vi "PTSAutoDaily.vi"() -> ()   [LabVIEW 2012]
uses:
  <vilib>/Utility/NIReport.llb/NI_report.lvclass
  <vilib>/addons/database/Connection.llb/DB Tools Open Connec (Path).vi
  <vilib>/addons/database/Connection.llb/Conn Execute.vi
  <vilib>/addons/database/Recordset.llb/Rec Fetch Recordset Data (R).vi
  <vilib>/addons/database/Recordset.llb/Rec Destroy - Connection.vi
  <vilib>/Utility/NIReport.llb/Append Text Table to Report (wrap).vi
  <vilib>/addons/database/_DB Variant To Data/Database Variant To Data.xnode
  <vilib>/addons/database/NI_Database_API.lvlib
  <vilib>/Utility/NIReport.llb/Excel/NI_Excel.lvclass
  <vilib>/addons/_office/NI_ReportGenerationToolkit.lvlib
panel:
  in  "Report Template":path=path "O:/Monitor/Report/PTSDailyReport.xls"
  in  "Table Control":string[][](table)
  in  "Table Control 2":string[][](table)
  in  "Table Control 3":string[][](table)
  in  "Table Control 4":string[][](table)
  out "error out 4":errorcluster
  out "error out 6":errorcluster
  out "appended array 5":string[](array[string])
  out "recordset data 5":variant[][](array[variant])
  out "error out 5":errorcluster
  out "appended array 4":string[](array[string])
  out "recordset data 4":variant[][](array[variant])
  out "error out 3":errorcluster
  out "appended array 3":string[](array[string])
  out "recordset data 3":variant[][](array[variant])
  out "error out":errorcluster
  out "appended array":string[](array[string])
  out "recordset data":variant[][](array[variant])
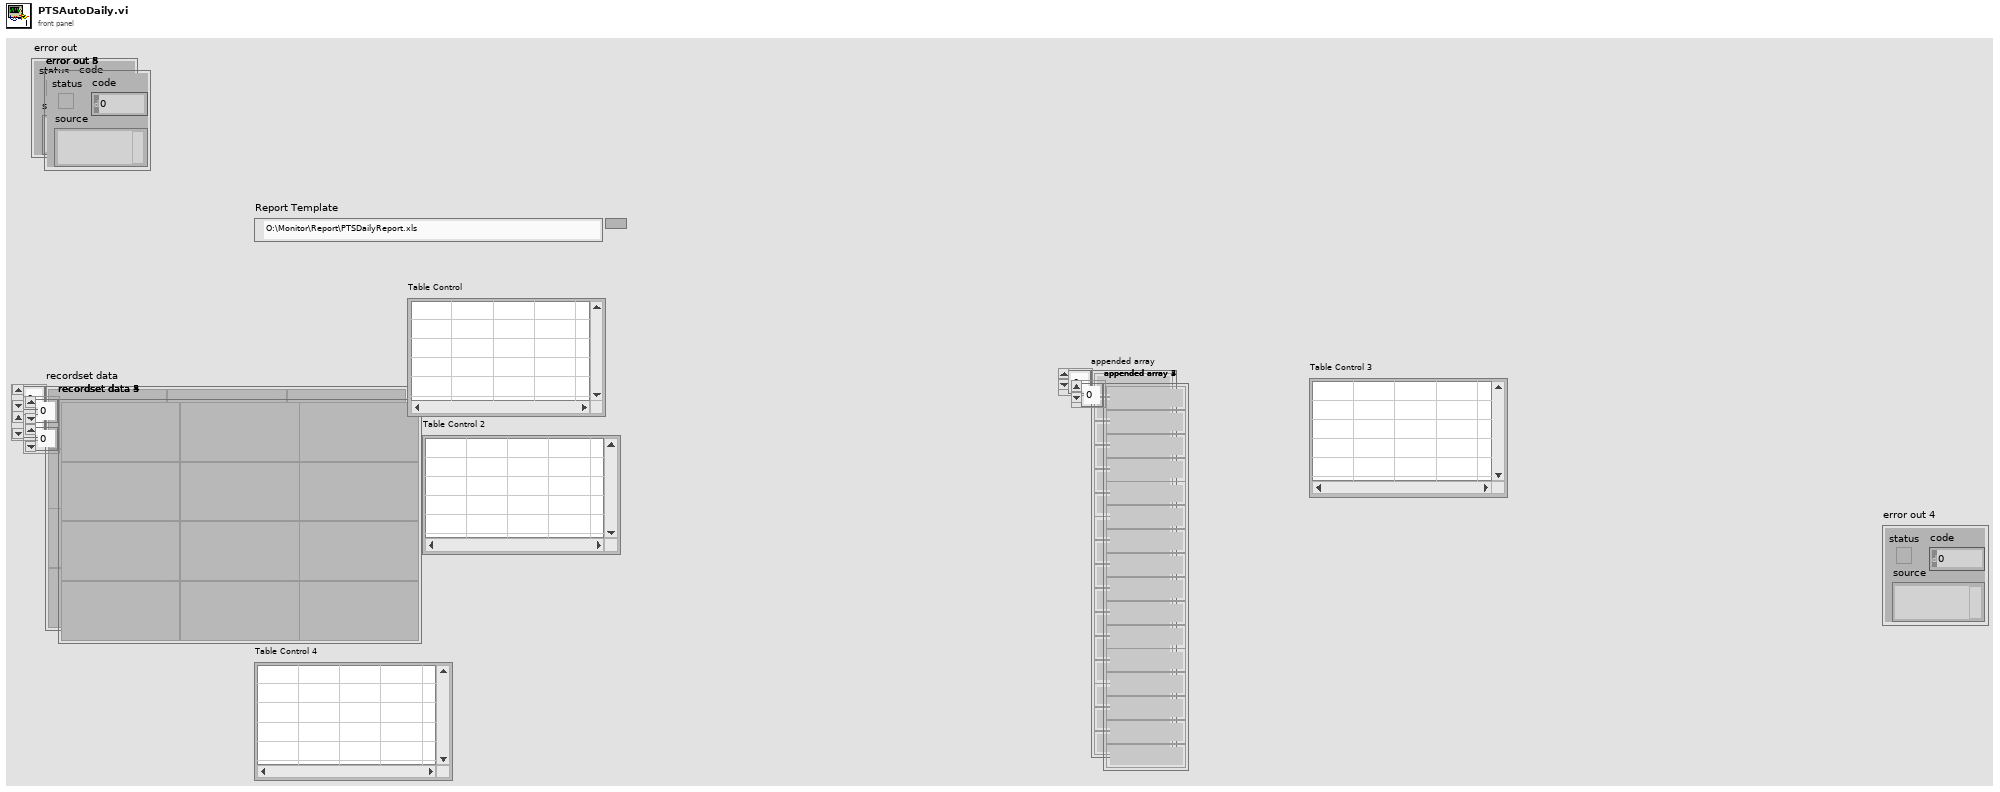
[diagram p1: front panel]
types:
  T1 = typedef "NI_Database_API.lvlib/Conn ObjectReference.ctl" = refnum<k1>
  T2 = typedef "NI_Database_API.lvlib/Rec ObjectReference.ctl" = refnum<k1>
  T3 = enum16{"Standard Report", "HTML", "Word", "Excel"}
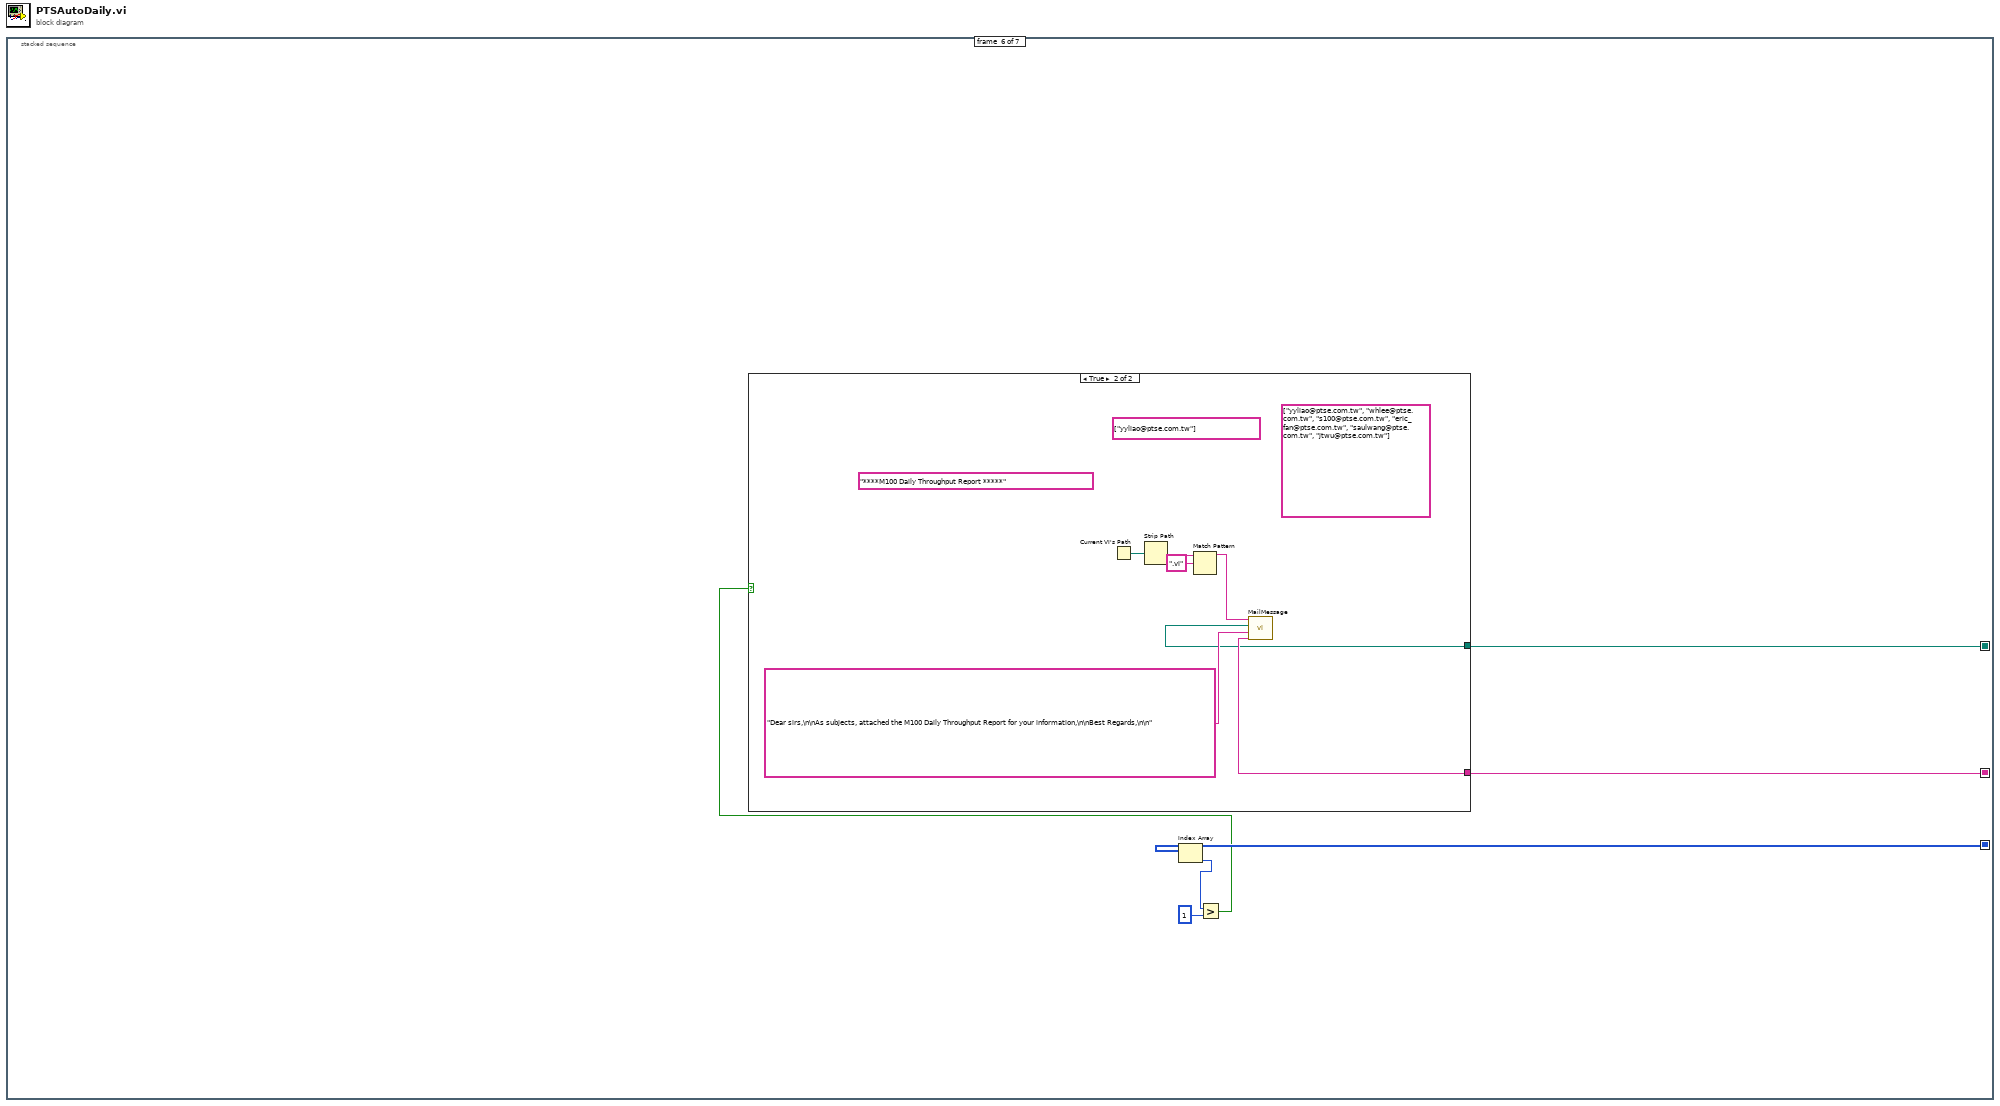
[diagram p0: block diagram]
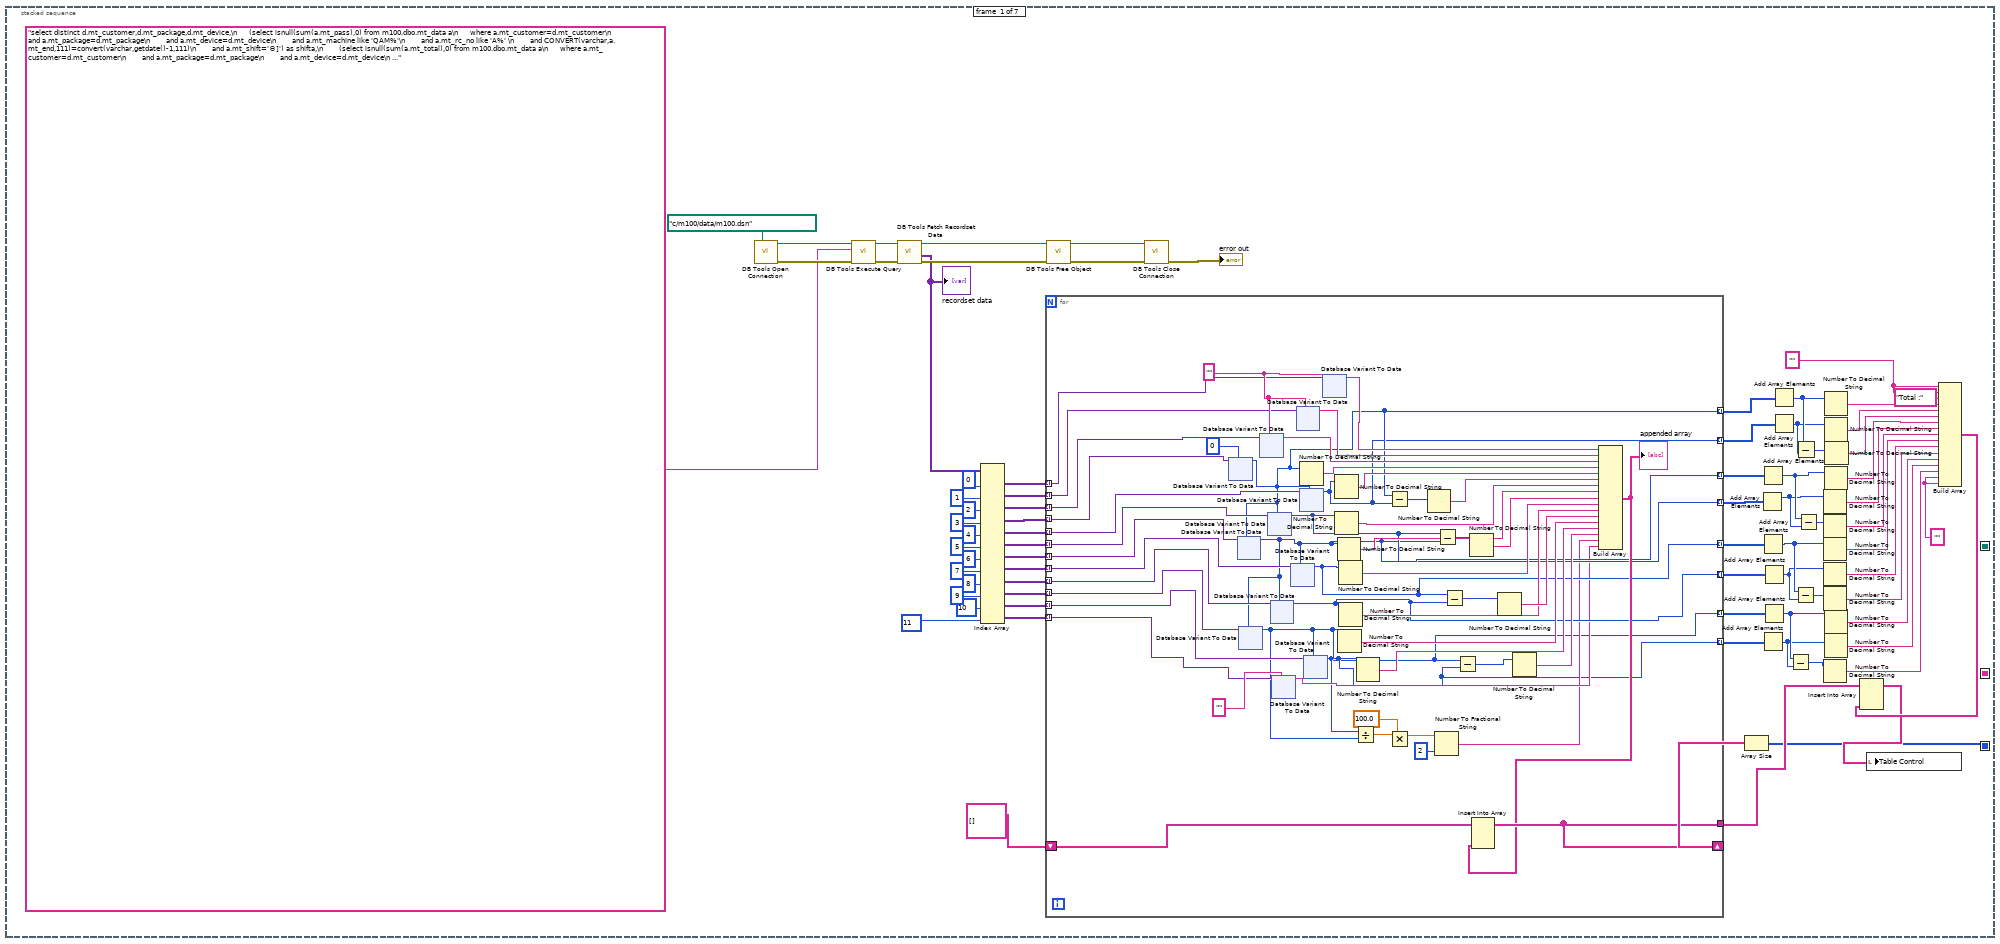
[diagram p2: hidden frame]
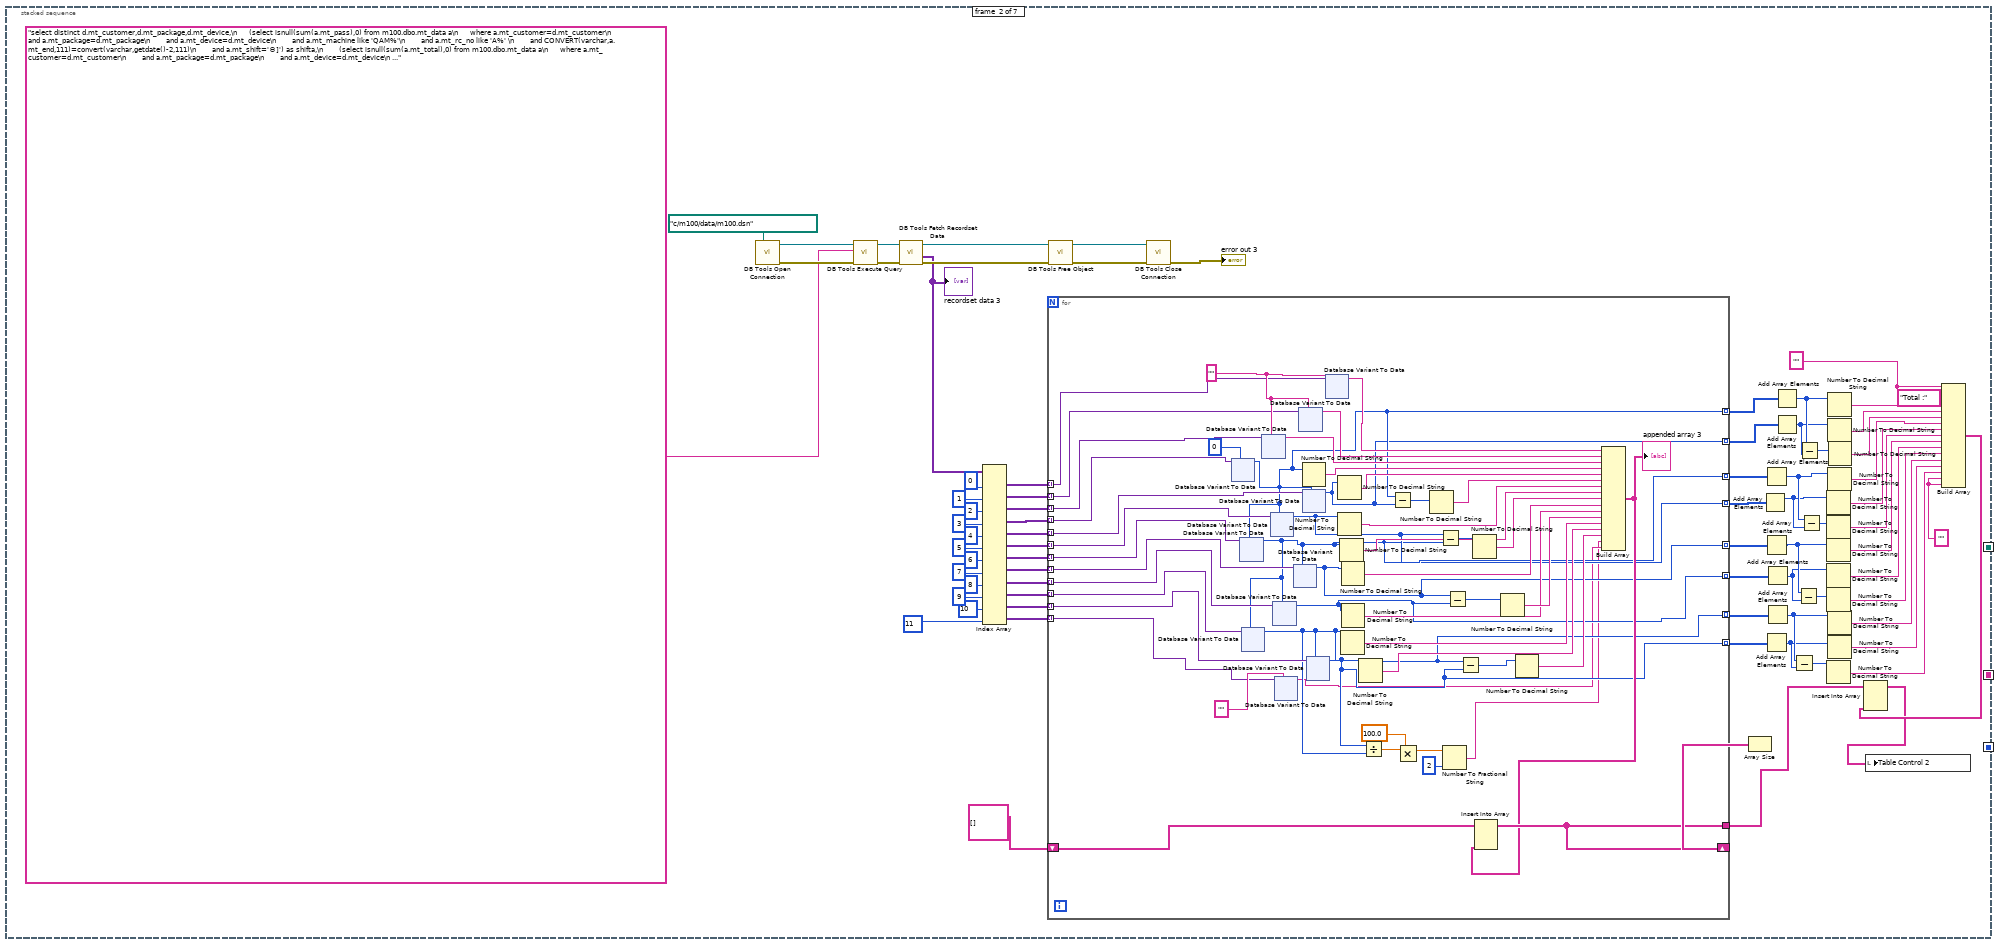
[diagram p3: hidden frame]
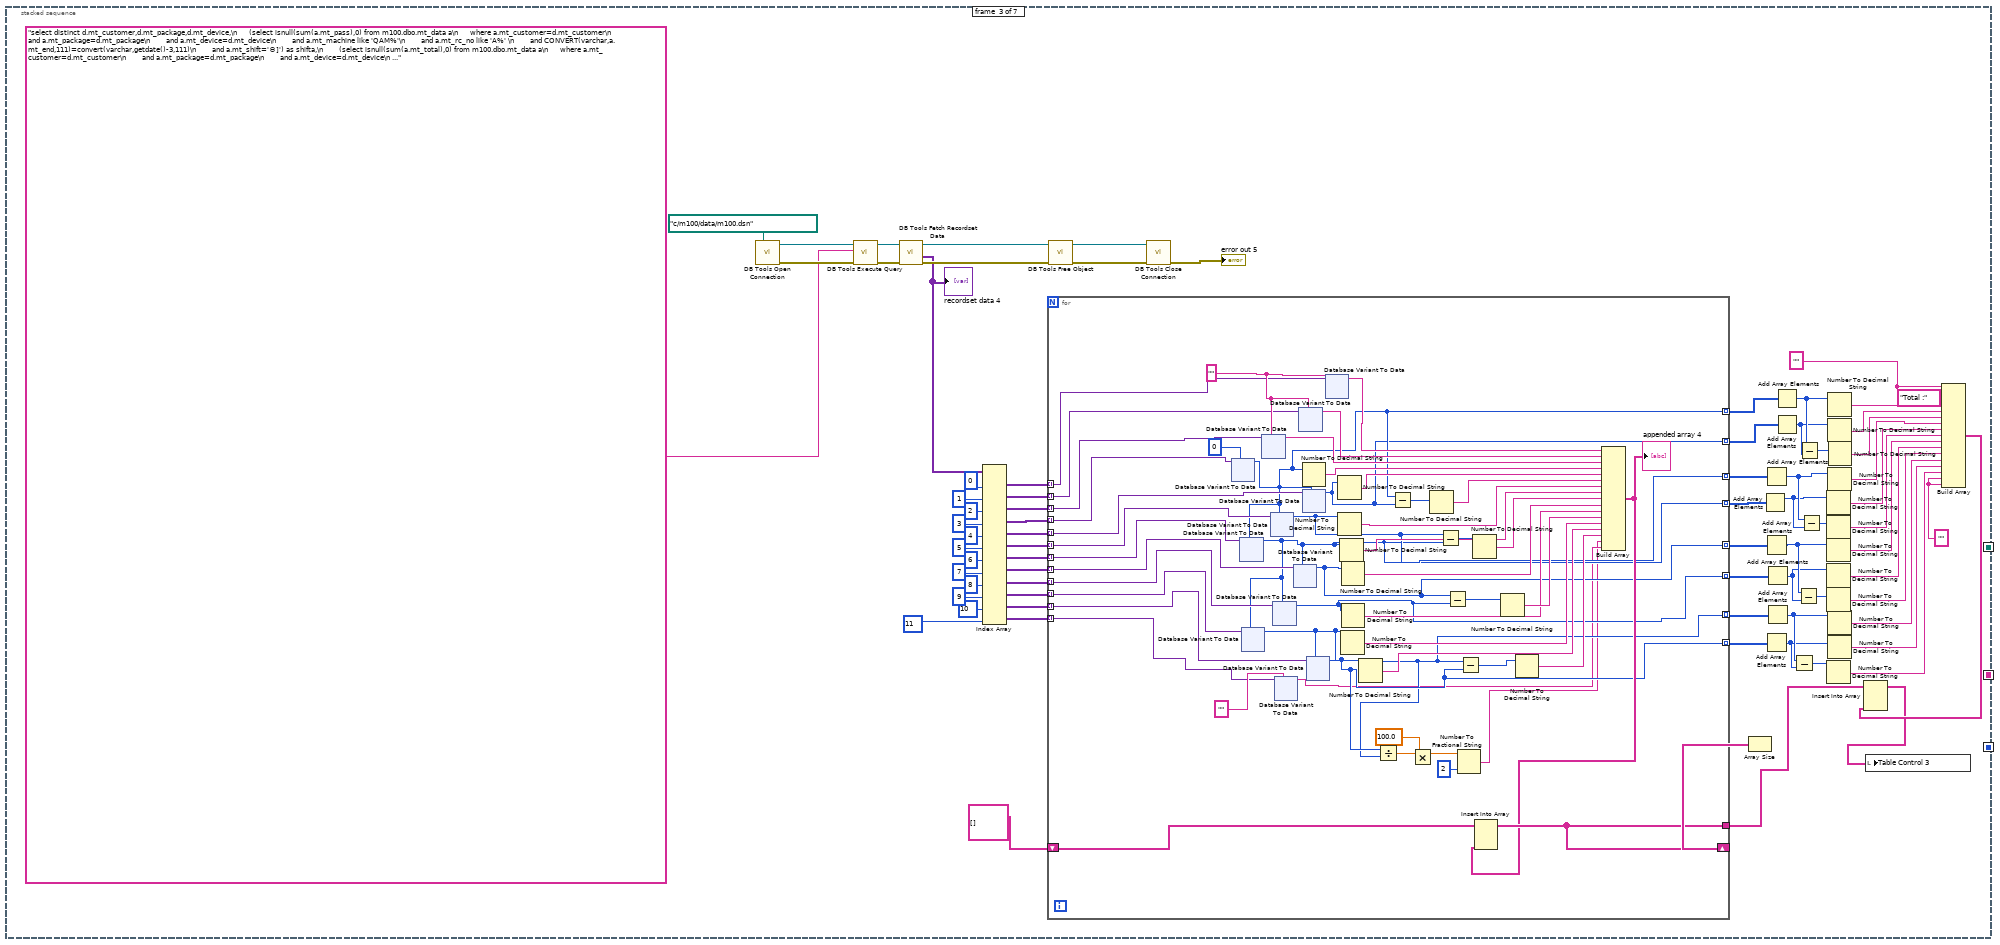
[diagram p4: hidden frame]
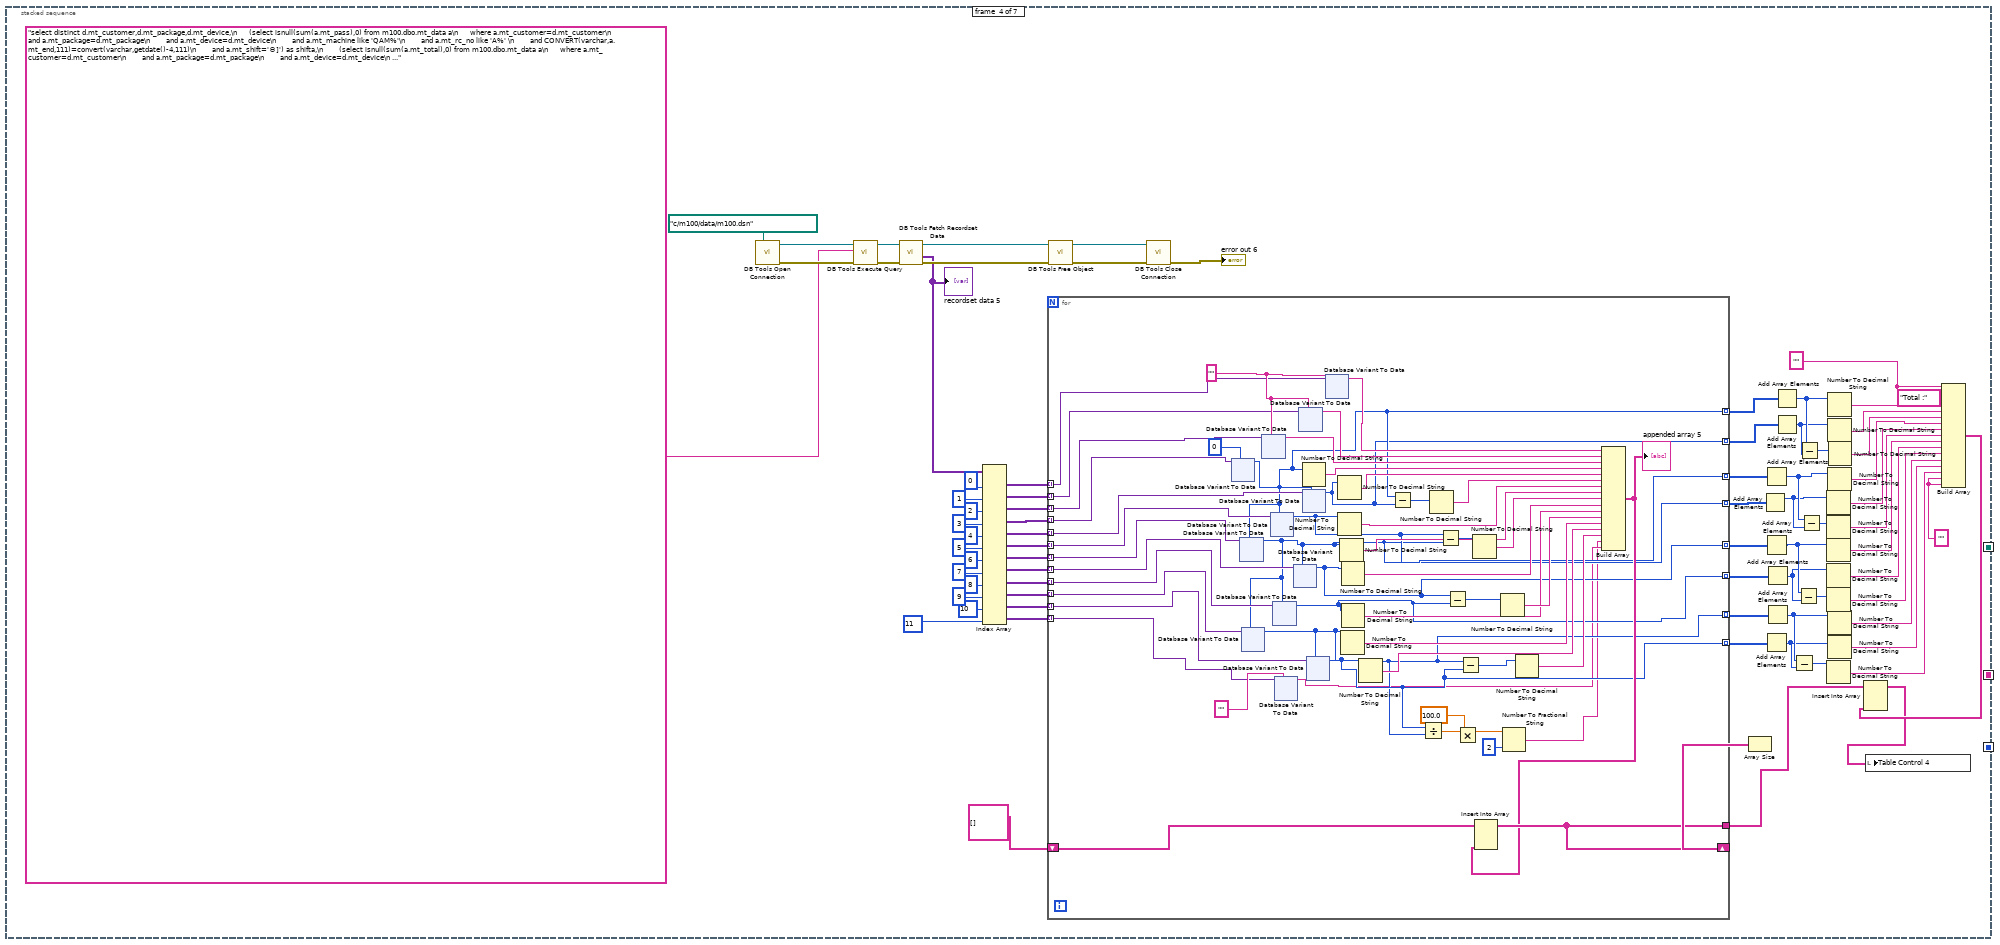
[diagram p5: hidden frame]
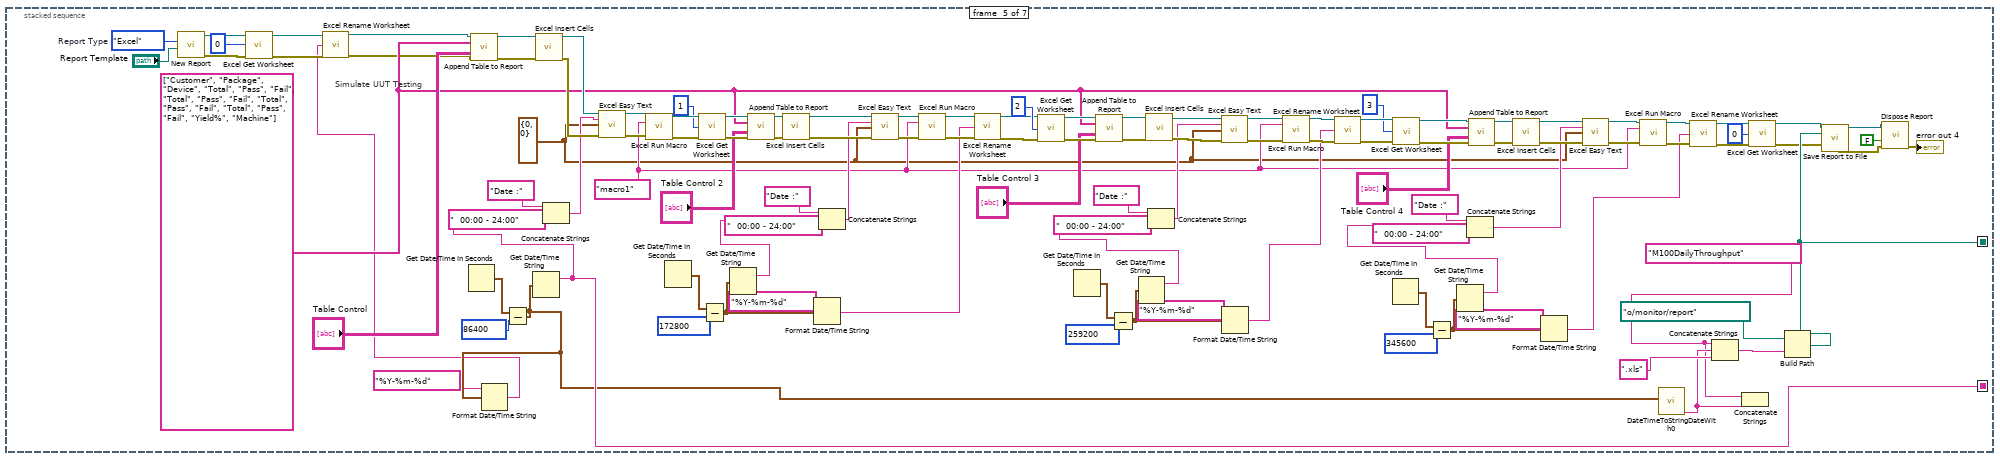
[diagram p6: hidden frame]
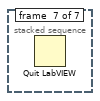
[diagram p8: hidden frame]
diagram:
  n1 = stacked-sequence {
    seq-local: [_ _ _ _ w2139 _ _] -> [_ _ _ _ _ w2163 _]
    seq-local: [_ _ _ _ w2138 _ _] -> [_ _ _ _ _ w2162 _]
    seq-local: [w2 _ _ _ _ _ _] -> [_ _ _ _ _ w2161 _]
    frame #0 {
      w1 = ""
      w37 = ""
      n2 = call-poly <vilib>:"DB Tools Open Connection.vi"("connection information"=path "c:/m100/data/m100.dsn") -> ("error out"=w72:errorcluster, "connection reference"=w76:T1)  [unwired: 7 in]
      n3 = call-poly <vilib>:"DB Tools Execute Query.vi"("error in (no error)"=w72, "SQL query"="select distinct d.mt_customer,d.mt_package,d.mt_device,\n      (select isnull(sum(a.mt_pass),0) from m100.dbo.mt_data a\n      where a.mt_customer=d.mt_customer\n        and a.mt_package=d.mt_package\n        and a.mt_device=d.mt_device\n        and a.mt_machine like 'QAM%'\n        and a.mt_rc_no like 'A%' \n        and CONVERT(varchar,a.mt_end,111)=convert(varchar,getdate()-1,111)\n        and a.mt_shift='©]') as shifta,\n        (select isnull(sum(a.mt_total),0) from m100.dbo.mt_data a\n      where a.mt_customer=d.mt_customer\n        and a.mt_package=d.mt_package\n        and a.mt_device=d.mt_device\n        and a.mt_machine like 'QAM%'\n        and a.mt_rc_no like 'A%' \n        and CONVERT(varchar,a.mt_end,111)=convert(varchar,getdate()-1,111)\n        and a.mt_shift='©]') as shifta1,\n        (select isnull(sum(b.mt_pass),0) from m100.dbo.mt_data b\n      where b.mt_customer=d.mt_customer\n        and b.mt_package=d.mt_package\n       and b.mt_device=d.mt_device\n        and b.mt_machine like 'QAM%'\n        and b.mt_rc_no like 'A%' \n        and CONVERT(varchar,b.mt_end,111)=convert(varchar,getdate()-1,111)\n        and b.mt_shift='¦­') as shiftb,\n        (select isnull(sum(b.mt_total),0) from m100.dbo.mt_data b\n      where b.mt_customer=d.mt_customer\n        and b.mt_package=d.mt_package\n        and b.mt_device=d.mt_device\n        and b.mt_machine like 'QAM%'\n        and b.mt_rc_no like 'A%' \n        and CONVERT(varchar,b.mt_end,111)=convert(varchar,getdate()-1,111)\n        and b.mt_shift='¦­') as shiftb1,\n        (select isnull(sum(c.mt_pass),0) from m100.dbo.mt_data c\n      where c.mt_customer=d.mt_customer\n        and c.mt_package=d.mt_package\n        and c.mt_device=d.mt_device\n        and c.mt_machine like 'QAM%'\n        and c.mt_rc_no like 'A%' \n        and CONVERT(varchar,c.mt_end,111)=convert(varchar,getdate()-1,111)\n        and c.mt_shift='¤¤') as shiftc,\n        (select isnull(sum(c.mt_total),0) from m100.dbo.mt_data c\n      where c.mt_customer=d.mt_customer\n        and c.mt_package=d.mt_package\n        and c.mt_device=d.mt_device\n        and c.mt_machine like 'QAM%'\n        and c.mt_rc_no like 'A%' \n        and CONVERT(varchar,c.mt_end,111)=convert(varchar,getdate()-1,111)\n        and c.mt_shift='¤¤') as shiftc1,\n        SUM(mt_pass),SUM(mt_total),master.dbo.GetEntityNameFromDateToDate(d.mt_customer,d.mt_package,d.mt_device,CONVERT(varchar,GETDATE()-1,111),CONVERT(varchar,GETDATE()-1,111))\n  FROM [m100].[dbo].[mt_data] d\n  WHERE d.mt_machine like 'QAM%'\n    AND CONVERT(varchar,d.mt_end,111)=convert(varchar,getdate()-1,111)\n    and d.mt_pass > 0 and d.mt_rc_no like 'A%'\n      group by d.mt_customer,d.mt_package,d.mt_device", "connection reference"=w76) -> ("error out"=w71:errorcluster, "recordset reference"=w75:T2)  [unwired: 5 in]
      n4 = call-poly <vilib>:"DB Tools Fetch Recordset Data.vi"("error in (no error)"=w71, "recordset reference"=w75) -> ("error out"=w70:errorcluster, "recordset data"=w40:variant[][], "recordset reference out"=w74:T2)  [unwired: 3 in]
      "recordset data" <- w40
      n5 = Index Array(array=w40, index (col) #1=0 ("index (row)"), index (col) #2=1 ("index (col)"), index (col) #3=2 ("disabled index (col)"), index (col) #4=3 ("index (col)"), index (col) #5=4 ("index (col)"), index (col) #6=5 ("index (col)"), index (col) #7=6 ("index (col)"), index (col) #8=7 ("index (col)"), index (col) #9=8 ("index (col)"), index (col) #10=9 ("index (col)"), index (col) #11=10 ("index (col)"), index (col) #12=11 ("index (col)")) -> (element #1=w44:variant[], element #2=w43:variant[], element #3=w57:variant[], element #4=w56:variant[], element #5=w55:variant[], element #6=w54:variant[], element #7=w53:variant[], element #8=w52:variant[], element #9=w51:variant[], element #10=w50:variant[], element #11=w49:variant[], element #12=w48:variant[])  [unwired: 12 in]
      n6 = for {
        tunnel: w57 -> [w102] mode=indexing
        tunnel: w56 -> [w101] mode=indexing
        tunnel: w55 -> [w100] mode=indexing
        tunnel: w54 -> [w99] mode=indexing
        tunnel: w53 -> [w98] mode=indexing
        tunnel: w52 -> [w97] mode=indexing
        tunnel: w51 -> [w96] mode=indexing
        tunnel: w50 -> [w95] mode=indexing
        tunnel: w49 -> [w94] mode=indexing
        tunnel: w48 -> [w93] mode=indexing
        tunnel: [w128] -> w30
        shift-right: [w128] -> w46
        shift-left: string[][] [] ("array") -> [w127]
        tunnel: w44 -> [w104] mode=indexing
        tunnel: w43 -> [w103] mode=indexing
        tunnel: [w91] -> w39 mode=indexing
        tunnel: [w90] -> w38 mode=indexing
        tunnel: [w89] -> w28 mode=indexing
        tunnel: [w88] -> w27 mode=indexing
        tunnel: [w87] -> w19 mode=indexing
        tunnel: [w86] -> w18 mode=indexing
        tunnel: [w78] -> w11 mode=indexing
        tunnel: [w79] -> w10 mode=indexing
        w126 = ""
        n7 = xnode "Database Variant To Data"("database variant"=w101, "type"=0) -> ("data"=w91:i32)  [unwired: 1 in, 1 out]
        n8 = xnode "Database Variant To Data"("database variant"=w98, "type"=w91) -> ("data"=w88:i32)  [unwired: 1 in, 1 out]
        n9 = xnode "Database Variant To Data"("database variant"=w95, "type"=w88) -> ("data"=w78:i32)  [unwired: 1 in, 1 out]
        n10 = xnode "Database Variant To Data"("database variant"=w102, "type"=w126) -> ("data"=w110:string)  [unwired: 1 in, 1 out]
        n11 = xnode "Database Variant To Data"("database variant"=w99, "type"=w91) -> ("data"=w89:i32)  [unwired: 1 in, 1 out]
        n12 = xnode "Database Variant To Data"("database variant"=w96, "type"=w88) -> ("data"=w86:i32)  [unwired: 1 in, 1 out]
        n13 = xnode "Database Variant To Data"("database variant"=w93, "type"="") -> ("data"=w81:string)  [unwired: 1 in, 1 out]
        n14 = xnode "Database Variant To Data"("database variant"=w97, "type"=w88) -> ("data"=w87:i32)  [unwired: 1 in, 1 out]
        n15 = xnode "Database Variant To Data"("database variant"=w103, "type"=w126) -> ("data"=w107:string)  [unwired: 1 in, 1 out]
        n16 = Number To Decimal String(number=w91) -> (decimal integer string=w109:string)  [unwired: 1 in]
        n17 = xnode "Database Variant To Data"("database variant"=w100, "type"=w91) -> ("data"=w90:i32)  [unwired: 1 in, 1 out]
        n18 = xnode "Database Variant To Data"("database variant"=w94, "type"=w78) -> ("data"=w79:i32)  [unwired: 1 in, 1 out]
        n19 = xnode "Database Variant To Data"("database variant"=w104, "type"=w126) -> ("data"=w111:string)  [unwired: 1 in, 1 out]
        n20 = Number To Decimal String(number=w90) -> (decimal integer string=w108:string)  [unwired: 1 in]
        n21 = Number To Decimal String(number=w89) -> (decimal integer string=w124:string)  [unwired: 1 in]
        n22 = Number To Decimal String(number=w88) -> (decimal integer string=w123:string)  [unwired: 1 in]
        n23 = Number To Decimal String(number=w78) -> (decimal integer string=w118:string)  [unwired: 1 in]
        n24 = Number To Decimal String(number=w87) -> (decimal integer string=w114:string)  [unwired: 1 in]
        n25 = Number To Decimal String(number=w86) -> (decimal integer string=w115:string)  [unwired: 1 in]
        n26 = Divide(x=w79, y=w78) -> (x/y=w85:dbl)
        n27 = Number To Decimal String(number=w79) -> (decimal integer string=w119:string)  [unwired: 1 in]
        n28 = Subtract(x=w91, y=w90) -> (x-y=w106:i32)
        n29 = Multiply(x=w85, y=100.0) -> (x*y=w83:dbl)
        n30 = Number To Decimal String(number=w106) -> (decimal integer string=w105:string)  [unwired: 1 in]
        n31 = Number To Fractional String(number=w83, precision (6)=i16 2) -> (F-format string=w80:string)  [unwired: 2 in]
        n32 = Subtract(x=w89, y=w88) -> (x-y=w113:i32)
        n33 = Subtract(x=w87, y=w86) -> (x-y=w117:i32)
        n34 = Subtract(x=w78, y=w79) -> (x-y=w121:i32)
        n35 = Number To Decimal String(number=w113) -> (decimal integer string=w112:string)  [unwired: 1 in]
        n36 = Number To Decimal String(number=w117) -> (decimal integer string=w116:string)  [unwired: 1 in]
        n37 = Number To Decimal String(number=w121) -> (decimal integer string=w120:string)  [unwired: 1 in]
        n38 = Build Array(w111, w107, w110, w109, w108, w105, w124, w123, w112, w114, w115, w116, w118, w119, w120, w80, w81) -> (w92:string[])
        "appended array" <- w92
        n39 = Insert Into Array(array=w127, new element=w92) -> (w128:string[][])  [unwired: 2 in]
      }
      n40 = call-poly <vilib>:"DB Tools Free Object.vi"("error in (no error)"=w70, "recordset reference"=w74) -> ("error out"=w69:errorcluster, "connection reference"=w73:T1)  [unwired: 8 in]
      n41 = call <vilib>:"DB Tools Close Connection.vi"("error in (no error)"=w69, "connection reference"=w73) -> ("error out"=→"error out":errorcluster)  [unwired: 5 in]
      n42 = Array Size(array=w46) -> (size(s)=w2:i32[])
      n43 = Add Array Elements(numeric array=w27) -> (sum=w22:i32)
      n44 = Add Array Elements(numeric array=w28) -> (sum=w23:i32)
      n45 = Add Array Elements(numeric array=w19) -> (sum=w15:i32)
      n46 = Add Array Elements(numeric array=w10) -> (sum=w8:i32)
      n47 = Add Array Elements(numeric array=w18) -> (sum=w14:i32)
      n48 = Add Array Elements(numeric array=w11) -> (sum=w9:i32)
      n49 = Add Array Elements(numeric array=w39) -> (sum=w34:i32)
      n50 = Add Array Elements(numeric array=w38) -> (sum=w33:i32)
      n51 = Subtract(x=w9, y=w8) -> (x-y=w7:i32)
      n52 = Subtract(x=w15, y=w14) -> (x-y=w12:i32)
      n53 = Subtract(x=w34, y=w33) -> (x-y=w26:i32)
      n54 = Subtract(x=w23, y=w22) -> (x-y=w20:i32)
      n55 = Number To Decimal String(number=w22) -> (decimal integer string=w24:string)  [unwired: 1 in]
      n56 = Number To Decimal String(number=w20) -> (decimal integer string=w21:string)  [unwired: 1 in]
      n57 = Number To Decimal String(number=w15) -> (decimal integer string=w17:string)  [unwired: 1 in]
      n58 = Number To Decimal String(number=w14) -> (decimal integer string=w16:string)  [unwired: 1 in]
      n59 = Number To Decimal String(number=w12) -> (decimal integer string=w13:string)  [unwired: 1 in]
      n60 = Number To Decimal String(number=w7) -> (decimal integer string=w4:string)  [unwired: 1 in]
      n61 = Number To Decimal String(number=w34) -> (decimal integer string=w36:string)  [unwired: 1 in]
      n62 = Number To Decimal String(number=w33) -> (decimal integer string=w35:string)  [unwired: 1 in]
      n63 = Number To Decimal String(number=w23) -> (decimal integer string=w25:string)  [unwired: 1 in]
      n64 = Number To Decimal String(number=w9) -> (decimal integer string=w6:string)  [unwired: 1 in]
      n65 = Number To Decimal String(number=w8) -> (decimal integer string=w5:string)  [unwired: 1 in]
      n66 = Number To Decimal String(number=w26) -> (decimal integer string=w32:string)  [unwired: 1 in]
      n67 = Build Array(w37, w37, "Total :" ("element"), w36, w35, w32, w25, w24, w21, w17, w16, w13, w6, w5, w4, w1, w1) -> (w31:string[])
      n68 = Insert Into Array(array=w30, new element=w31) -> (w29:string[][])  [unwired: 2 in]
      n69 = local write "Table Control"(w29) -> ()
    }
    frame #1 {
      w513 = ""
      w548 = ""
      n70 = call-poly <vilib>:"DB Tools Open Connection.vi"("connection information"=path "c:/m100/data/m100.dsn") -> ("error out"=w583:errorcluster, "connection reference"=w587:T1)  [unwired: 7 in]
      n71 = call-poly <vilib>:"DB Tools Execute Query.vi"("error in (no error)"=w583, "SQL query"="select distinct d.mt_customer,d.mt_package,d.mt_device,\n      (select isnull(sum(a.mt_pass),0) from m100.dbo.mt_data a\n      where a.mt_customer=d.mt_customer\n        and a.mt_package=d.mt_package\n        and a.mt_device=d.mt_device\n        and a.mt_machine like 'QAM%'\n        and a.mt_rc_no like 'A%' \n        and CONVERT(varchar,a.mt_end,111)=convert(varchar,getdate()-2,111)\n        and a.mt_shift='©]') as shifta,\n        (select isnull(sum(a.mt_total),0) from m100.dbo.mt_data a\n      where a.mt_customer=d.mt_customer\n        and a.mt_package=d.mt_package\n        and a.mt_device=d.mt_device\n        and a.mt_machine like 'QAM%'\n        and a.mt_rc_no like 'A%' \n        and CONVERT(varchar,a.mt_end,111)=convert(varchar,getdate()-2,111)\n        and a.mt_shift='©]') as shifta1,\n        (select isnull(sum(b.mt_pass),0) from m100.dbo.mt_data b\n      where b.mt_customer=d.mt_customer\n        and b.mt_package=d.mt_package\n       and b.mt_device=d.mt_device\n        and b.mt_machine like 'QAM%'\n        and b.mt_rc_no like 'A%' \n        and CONVERT(varchar,b.mt_end,111)=convert(varchar,getdate()-2,111)\n        and b.mt_shift='¦­') as shiftb,\n        (select isnull(sum(b.mt_total),0) from m100.dbo.mt_data b\n      where b.mt_customer=d.mt_customer\n        and b.mt_package=d.mt_package\n        and b.mt_device=d.mt_device\n        and b.mt_machine like 'QAM%'\n        and b.mt_rc_no like 'A%' \n        and CONVERT(varchar,b.mt_end,111)=convert(varchar,getdate()-2,111)\n        and b.mt_shift='¦­') as shiftb1,\n        (select isnull(sum(c.mt_pass),0) from m100.dbo.mt_data c\n      where c.mt_customer=d.mt_customer\n        and c.mt_package=d.mt_package\n        and c.mt_device=d.mt_device\n        and c.mt_machine like 'QAM%'\n        and c.mt_rc_no like 'A%' \n        and CONVERT(varchar,c.mt_end,111)=convert(varchar,getdate()-2,111)\n        and c.mt_shift='¤¤') as shiftc,\n        (select isnull(sum(c.mt_total),0) from m100.dbo.mt_data c\n      where c.mt_customer=d.mt_customer\n        and c.mt_package=d.mt_package\n        and c.mt_device=d.mt_device\n        and c.mt_machine like 'QAM%'\n        and c.mt_rc_no like 'A%' \n        and CONVERT(varchar,c.mt_end,111)=convert(varchar,getdate()-2,111)\n        and c.mt_shift='¤¤') as shiftc1,\n        SUM(mt_pass),SUM(mt_total),master.dbo.GetEntityNameFromDateToDate(d.mt_customer,d.mt_package,d.mt_device,CONVERT(varchar,GETDATE()-2,111),CONVERT(varchar,GETDATE()-2,111))\n  FROM [m100].[dbo].[mt_data] d\n  WHERE  d.mt_machine like 'QAM%'\n    AND CONVERT(varchar,d.mt_end,111)=convert(varchar,getdate()-2,111)\n    and d.mt_pass > 0 and d.mt_rc_no like 'A%'\n      group by d.mt_customer,d.mt_package,d.mt_device", "connection reference"=w587) -> ("error out"=w582:errorcluster, "recordset reference"=w586:T2)  [unwired: 5 in]
      n72 = call-poly <vilib>:"DB Tools Fetch Recordset Data.vi"("error in (no error)"=w582, "recordset reference"=w586) -> ("error out"=w581:errorcluster, "recordset data"=w551:variant[][], "recordset reference out"=w585:T2)  [unwired: 3 in]
      "recordset data 3" <- w551
      n73 = Index Array(array=w551, index (col) #1=0 ("index (row)"), index (col) #2=1 ("index (col)"), index (col) #3=2 ("disabled index (col)"), index (col) #4=3 ("index (col)"), index (col) #5=4 ("index (col)"), index (col) #6=5 ("index (col)"), index (col) #7=6 ("index (col)"), index (col) #8=7 ("index (col)"), index (col) #9=8 ("index (col)"), index (col) #10=9 ("index (col)"), index (col) #11=10 ("index (col)"), index (col) #12=11 ("index (col)")) -> (element #1=w555:variant[], element #2=w554:variant[], element #3=w568:variant[], element #4=w567:variant[], element #5=w566:variant[], element #6=w565:variant[], element #7=w564:variant[], element #8=w563:variant[], element #9=w562:variant[], element #10=w561:variant[], element #11=w560:variant[], element #12=w559:variant[])  [unwired: 12 in]
      n74 = for {
        tunnel: w568 -> [w613] mode=indexing
        tunnel: w567 -> [w612] mode=indexing
        tunnel: w566 -> [w611] mode=indexing
        tunnel: w565 -> [w610] mode=indexing
        tunnel: w564 -> [w609] mode=indexing
        tunnel: w563 -> [w608] mode=indexing
        tunnel: w562 -> [w607] mode=indexing
        tunnel: w561 -> [w606] mode=indexing
        tunnel: w560 -> [w605] mode=indexing
        tunnel: w559 -> [w604] mode=indexing
        tunnel: [w639] -> w541
        shift-right: [w639] -> w557
        shift-left: string[][] [] ("array") -> [w638]
        tunnel: w555 -> [w615] mode=indexing
        tunnel: w554 -> [w614] mode=indexing
        tunnel: [w602] -> w550 mode=indexing
        tunnel: [w601] -> w549 mode=indexing
        tunnel: [w600] -> w539 mode=indexing
        tunnel: [w599] -> w538 mode=indexing
        tunnel: [w598] -> w530 mode=indexing
        tunnel: [w597] -> w529 mode=indexing
        tunnel: [w591] -> w522 mode=indexing
        tunnel: [w592] -> w521 mode=indexing
        w637 = ""
        n75 = xnode "Database Variant To Data"("database variant"=w612, "type"=0) -> ("data"=w602:i32)  [unwired: 1 in, 1 out]
        n76 = xnode "Database Variant To Data"("database variant"=w609, "type"=w602) -> ("data"=w599:i32)  [unwired: 1 in, 1 out]
        n77 = xnode "Database Variant To Data"("database variant"=w606, "type"=w599) -> ("data"=w591:i32)  [unwired: 1 in, 1 out]
        n78 = xnode "Database Variant To Data"("database variant"=w613, "type"=w637) -> ("data"=w621:string)  [unwired: 1 in, 1 out]
        n79 = xnode "Database Variant To Data"("database variant"=w610, "type"=w602) -> ("data"=w600:i32)  [unwired: 1 in, 1 out]
        n80 = xnode "Database Variant To Data"("database variant"=w607, "type"=w599) -> ("data"=w597:i32)  [unwired: 1 in, 1 out]
        n81 = xnode "Database Variant To Data"("database variant"=w604, "type"="") -> ("data"=w590:string)  [unwired: 1 in, 1 out]
        n82 = xnode "Database Variant To Data"("database variant"=w608, "type"=w599) -> ("data"=w598:i32)  [unwired: 1 in, 1 out]
        n83 = xnode "Database Variant To Data"("database variant"=w614, "type"=w637) -> ("data"=w618:string)  [unwired: 1 in, 1 out]
        n84 = Number To Decimal String(number=w602) -> (decimal integer string=w620:string)  [unwired: 1 in]
        n85 = xnode "Database Variant To Data"("database variant"=w611, "type"=w602) -> ("data"=w601:i32)  [unwired: 1 in, 1 out]
        n86 = xnode "Database Variant To Data"("database variant"=w605, "type"=w591) -> ("data"=w592:i32)  [unwired: 1 in, 1 out]
        n87 = xnode "Database Variant To Data"("database variant"=w615, "type"=w637) -> ("data"=w622:string)  [unwired: 1 in, 1 out]
        n88 = Number To Decimal String(number=w601) -> (decimal integer string=w619:string)  [unwired: 1 in]
        n89 = Number To Decimal String(number=w600) -> (decimal integer string=w635:string)  [unwired: 1 in]
        n90 = Number To Decimal String(number=w599) -> (decimal integer string=w634:string)  [unwired: 1 in]
        n91 = Number To Decimal String(number=w591) -> (decimal integer string=w629:string)  [unwired: 1 in]
        n92 = Number To Decimal String(number=w598) -> (decimal integer string=w625:string)  [unwired: 1 in]
        n93 = Number To Decimal String(number=w597) -> (decimal integer string=w626:string)  [unwired: 1 in]
        n94 = Number To Decimal String(number=w592) -> (decimal integer string=w630:string)  [unwired: 1 in]
        n95 = Divide(x=w592, y=w591) -> (x/y=w596:dbl)
        n96 = Subtract(x=w602, y=w601) -> (x-y=w617:i32)
        n97 = Multiply(x=w596, y=100.0) -> (x*y=w594:dbl)
        n98 = Number To Decimal String(number=w617) -> (decimal integer string=w616:string)  [unwired: 1 in]
        n99 = Subtract(x=w600, y=w599) -> (x-y=w624:i32)
        n100 = Number To Fractional String(number=w594, precision (6)=i16 2) -> (F-format string=w589:string)  [unwired: 2 in]
        n101 = Subtract(x=w598, y=w597) -> (x-y=w628:i32)
        n102 = Subtract(x=w591, y=w592) -> (x-y=w632:i32)
        n103 = Number To Decimal String(number=w624) -> (decimal integer string=w623:string)  [unwired: 1 in]
        n104 = Number To Decimal String(number=w628) -> (decimal integer string=w627:string)  [unwired: 1 in]
        n105 = Number To Decimal String(number=w632) -> (decimal integer string=w631:string)  [unwired: 1 in]
        n106 = Build Array(w622, w618, w621, w620, w619, w616, w635, w634, w623, w625, w626, w627, w629, w630, w631, w589, w590) -> (w603:string[])
        "appended array 3" <- w603
        n107 = Insert Into Array(array=w638, new element=w603) -> (w639:string[][])  [unwired: 2 in]
      }
      n108 = call-poly <vilib>:"DB Tools Free Object.vi"("error in (no error)"=w581, "recordset reference"=w585) -> ("error out"=w580:errorcluster, "connection reference"=w584:T1)  [unwired: 8 in]
      n109 = call <vilib>:"DB Tools Close Connection.vi"("error in (no error)"=w580, "connection reference"=w584) -> ("error out"=→"error out 3":errorcluster)  [unwired: 5 in]
      n110 = Array Size(array=w557) -> ()  [unwired: 1 out]
      n111 = Add Array Elements(numeric array=w538) -> (sum=w533:i32)
      n112 = Add Array Elements(numeric array=w539) -> (sum=w534:i32)
      n113 = Add Array Elements(numeric array=w530) -> (sum=w526:i32)
      n114 = Add Array Elements(numeric array=w521) -> (sum=w519:i32)
      n115 = Add Array Elements(numeric array=w529) -> (sum=w525:i32)
      n116 = Add Array Elements(numeric array=w522) -> (sum=w520:i32)
      n117 = Add Array Elements(numeric array=w550) -> (sum=w545:i32)
      n118 = Add Array Elements(numeric array=w549) -> (sum=w544:i32)
      n119 = Subtract(x=w520, y=w519) -> (x-y=w518:i32)
      n120 = Subtract(x=w526, y=w525) -> (x-y=w523:i32)
      n121 = Subtract(x=w545, y=w544) -> (x-y=w537:i32)
      n122 = Subtract(x=w534, y=w533) -> (x-y=w531:i32)
      n123 = Number To Decimal String(number=w533) -> (decimal integer string=w535:string)  [unwired: 1 in]
      n124 = Number To Decimal String(number=w531) -> (decimal integer string=w532:string)  [unwired: 1 in]
      n125 = Number To Decimal String(number=w526) -> (decimal integer string=w528:string)  [unwired: 1 in]
      n126 = Number To Decimal String(number=w525) -> (decimal integer string=w527:string)  [unwired: 1 in]
      n127 = Number To Decimal String(number=w523) -> (decimal integer string=w524:string)  [unwired: 1 in]
      n128 = Number To Decimal String(number=w518) -> (decimal integer string=w515:string)  [unwired: 1 in]
      n129 = Number To Decimal String(number=w545) -> (decimal integer string=w547:string)  [unwired: 1 in]
      n130 = Number To Decimal String(number=w544) -> (decimal integer string=w546:string)  [unwired: 1 in]
      n131 = Number To Decimal String(number=w534) -> (decimal integer string=w536:string)  [unwired: 1 in]
      n132 = Number To Decimal String(number=w520) -> (decimal integer string=w517:string)  [unwired: 1 in]
      n133 = Number To Decimal String(number=w519) -> (decimal integer string=w516:string)  [unwired: 1 in]
      n134 = Number To Decimal String(number=w537) -> (decimal integer string=w543:string)  [unwired: 1 in]
      n135 = Build Array(w548, w548, "Total :" ("element"), w547, w546, w543, w536, w535, w532, w528, w527, w524, w517, w516, w515, w513, w513) -> (w542:string[])
      n136 = Insert Into Array(array=w541, new element=w542) -> (w540:string[][])  [unwired: 2 in]
      n137 = local write "Table Control 2"(w540) -> ()
    }
    frame #2 {
      w1024 = ""
      w1059 = ""
      n138 = call-poly <vilib>:"DB Tools Open Connection.vi"("connection information"=path "c:/m100/data/m100.dsn") -> ("error out"=w1094:errorcluster, "connection reference"=w1098:T1)  [unwired: 7 in]
      n139 = call-poly <vilib>:"DB Tools Execute Query.vi"("error in (no error)"=w1094, "SQL query"="select distinct d.mt_customer,d.mt_package,d.mt_device,\n      (select isnull(sum(a.mt_pass),0) from m100.dbo.mt_data a\n      where a.mt_customer=d.mt_customer\n        and a.mt_package=d.mt_package\n        and a.mt_device=d.mt_device\n        and a.mt_machine like 'QAM%'\n        and a.mt_rc_no like 'A%' \n        and CONVERT(varchar,a.mt_end,111)=convert(varchar,getdate()-3,111)\n        and a.mt_shift='©]') as shifta,\n        (select isnull(sum(a.mt_total),0) from m100.dbo.mt_data a\n      where a.mt_customer=d.mt_customer\n        and a.mt_package=d.mt_package\n        and a.mt_device=d.mt_device\n        and a.mt_machine like 'QAM%'\n        and a.mt_rc_no like 'A%' \n        and CONVERT(varchar,a.mt_end,111)=convert(varchar,getdate()-3,111)\n        and a.mt_shift='©]') as shifta1,\n        (select isnull(sum(b.mt_pass),0) from m100.dbo.mt_data b\n      where b.mt_customer=d.mt_customer\n        and b.mt_package=d.mt_package\n       and b.mt_device=d.mt_device\n        and b.mt_machine like 'QAM%'\n        and b.mt_rc_no like 'A%' \n        and CONVERT(varchar,b.mt_end,111)=convert(varchar,getdate()-3,111)\n        and b.mt_shift='¦­') as shiftb,\n        (select isnull(sum(b.mt_total),0) from m100.dbo.mt_data b\n      where b.mt_customer=d.mt_customer\n        and b.mt_package=d.mt_package\n        and b.mt_device=d.mt_device\n        and b.mt_machine like 'QAM%'\n        and b.mt_rc_no like 'A%' \n        and CONVERT(varchar,b.mt_end,111)=convert(varchar,getdate()-3,111)\n        and b.mt_shift='¦­') as shiftb1,\n        (select isnull(sum(c.mt_pass),0) from m100.dbo.mt_data c\n      where c.mt_customer=d.mt_customer\n        and c.mt_package=d.mt_package\n        and c.mt_device=d.mt_device\n        and c.mt_machine like 'QAM%'\n        and c.mt_rc_no like 'A%' \n        and CONVERT(varchar,c.mt_end,111)=convert(varchar,getdate()-3,111)\n        and c.mt_shift='¤¤') as shiftc,\n        (select isnull(sum(c.mt_total),0) from m100.dbo.mt_data c\n      where c.mt_customer=d.mt_customer\n        and c.mt_package=d.mt_package\n        and c.mt_device=d.mt_device\n        and c.mt_machine like 'QAM%'\n        and c.mt_rc_no like 'A%' \n        and CONVERT(varchar,c.mt_end,111)=convert(varchar,getdate()-3,111)\n        and c.mt_shift='¤¤') as shiftc1,\n        SUM(mt_pass),SUM(mt_total),master.dbo.GetEntityNameFromDateToDate(d.mt_customer,d.mt_package,d.mt_device,CONVERT(varchar,GETDATE()-3,111),CONVERT(varchar,GETDATE()-3,111))\n  FROM [m100].[dbo].[mt_data] d\n  WHERE  d.mt_machine like 'QAM%'\n    AND CONVERT(varchar,d.mt_end,111)=convert(varchar,getdate()-3,111)\n    and d.mt_pass > 0 and d.mt_rc_no like 'A%'\n      group by d.mt_customer,d.mt_package,d.mt_device", "connection reference"=w1098) -> ("error out"=w1093:errorcluster, "recordset reference"=w1097:T2)  [unwired: 5 in]
      n140 = call-poly <vilib>:"DB Tools Fetch Recordset Data.vi"("error in (no error)"=w1093, "recordset reference"=w1097) -> ("error out"=w1092:errorcluster, "recordset data"=w1062:variant[][], "recordset reference out"=w1096:T2)  [unwired: 3 in]
      "recordset data 4" <- w1062
      n141 = Index Array(array=w1062, index (col) #1=0 ("index (row)"), index (col) #2=1 ("index (col)"), index (col) #3=2 ("disabled index (col)"), index (col) #4=3 ("index (col)"), index (col) #5=4 ("index (col)"), index (col) #6=5 ("index (col)"), index (col) #7=6 ("index (col)"), index (col) #8=7 ("index (col)"), index (col) #9=8 ("index (col)"), index (col) #10=9 ("index (col)"), index (col) #11=10 ("index (col)"), index (col) #12=11 ("index (col)")) -> (element #1=w1066:variant[], element #2=w1065:variant[], element #3=w1079:variant[], element #4=w1078:variant[], element #5=w1077:variant[], element #6=w1076:variant[], element #7=w1075:variant[], element #8=w1074:variant[], element #9=w1073:variant[], element #10=w1072:variant[], element #11=w1071:variant[], element #12=w1070:variant[])  [unwired: 12 in]
      n142 = for {
        tunnel: w1079 -> [w1124] mode=indexing
        tunnel: w1078 -> [w1123] mode=indexing
        tunnel: w1077 -> [w1122] mode=indexing
        tunnel: w1076 -> [w1121] mode=indexing
        tunnel: w1075 -> [w1120] mode=indexing
        tunnel: w1074 -> [w1119] mode=indexing
        tunnel: w1073 -> [w1118] mode=indexing
        tunnel: w1072 -> [w1117] mode=indexing
        tunnel: w1071 -> [w1116] mode=indexing
        tunnel: w1070 -> [w1115] mode=indexing
        tunnel: [w1150] -> w1052
        shift-right: [w1150] -> w1068
        shift-left: string[][] [] ("array") -> [w1149]
        tunnel: w1066 -> [w1126] mode=indexing
        tunnel: w1065 -> [w1125] mode=indexing
        tunnel: [w1113] -> w1061 mode=indexing
        tunnel: [w1112] -> w1060 mode=indexing
        tunnel: [w1111] -> w1050 mode=indexing
        tunnel: [w1110] -> w1049 mode=indexing
        tunnel: [w1109] -> w1041 mode=indexing
        tunnel: [w1108] -> w1040 mode=indexing
        tunnel: [w1102] -> w1033 mode=indexing
        tunnel: [w1103] -> w1032 mode=indexing
        w1148 = ""
        n143 = xnode "Database Variant To Data"("database variant"=w1123, "type"=0) -> ("data"=w1113:i32)  [unwired: 1 in, 1 out]
        n144 = xnode "Database Variant To Data"("database variant"=w1120, "type"=w1113) -> ("data"=w1110:i32)  [unwired: 1 in, 1 out]
        n145 = xnode "Database Variant To Data"("database variant"=w1117, "type"=w1110) -> ("data"=w1102:i32)  [unwired: 1 in, 1 out]
        n146 = xnode "Database Variant To Data"("database variant"=w1124, "type"=w1148) -> ("data"=w1132:string)  [unwired: 1 in, 1 out]
        n147 = xnode "Database Variant To Data"("database variant"=w1121, "type"=w1113) -> ("data"=w1111:i32)  [unwired: 1 in, 1 out]
        n148 = xnode "Database Variant To Data"("database variant"=w1118, "type"=w1110) -> ("data"=w1108:i32)  [unwired: 1 in, 1 out]
        n149 = xnode "Database Variant To Data"("database variant"=w1115, "type"="") -> ("data"=w1101:string)  [unwired: 1 in, 1 out]
        n150 = xnode "Database Variant To Data"("database variant"=w1119, "type"=w1110) -> ("data"=w1109:i32)  [unwired: 1 in, 1 out]
        n151 = xnode "Database Variant To Data"("database variant"=w1125, "type"=w1148) -> ("data"=w1129:string)  [unwired: 1 in, 1 out]
        n152 = Number To Decimal String(number=w1113) -> (decimal integer string=w1131:string)  [unwired: 1 in]
        n153 = xnode "Database Variant To Data"("database variant"=w1122, "type"=w1113) -> ("data"=w1112:i32)  [unwired: 1 in, 1 out]
        n154 = xnode "Database Variant To Data"("database variant"=w1116, "type"=w1102) -> ("data"=w1103:i32)  [unwired: 1 in, 1 out]
        n155 = xnode "Database Variant To Data"("database variant"=w1126, "type"=w1148) -> ("data"=w1133:string)  [unwired: 1 in, 1 out]
        n156 = Number To Decimal String(number=w1112) -> (decimal integer string=w1130:string)  [unwired: 1 in]
        n157 = Number To Decimal String(number=w1111) -> (decimal integer string=w1146:string)  [unwired: 1 in]
        n158 = Number To Decimal String(number=w1110) -> (decimal integer string=w1145:string)  [unwired: 1 in]
        n159 = Number To Decimal String(number=w1102) -> (decimal integer string=w1140:string)  [unwired: 1 in]
        n160 = Number To Decimal String(number=w1109) -> (decimal integer string=w1136:string)  [unwired: 1 in]
        n161 = Number To Decimal String(number=w1108) -> (decimal integer string=w1137:string)  [unwired: 1 in]
        n162 = Number To Decimal String(number=w1103) -> (decimal integer string=w1141:string)  [unwired: 1 in]
        n163 = Divide(x=w1103, y=w1102) -> (x/y=w1107:dbl)
        n164 = Subtract(x=w1113, y=w1112) -> (x-y=w1128:i32)
        n165 = Multiply(x=w1107, y=100.0) -> (x*y=w1105:dbl)
        n166 = Number To Decimal String(number=w1128) -> (decimal integer string=w1127:string)  [unwired: 1 in]
        n167 = Subtract(x=w1111, y=w1110) -> (x-y=w1135:i32)
        n168 = Subtract(x=w1109, y=w1108) -> (x-y=w1139:i32)
        n169 = Number To Fractional String(number=w1105, precision (6)=i16 2) -> (F-format string=w1100:string)  [unwired: 2 in]
        n170 = Subtract(x=w1102, y=w1103) -> (x-y=w1143:i32)
        n171 = Number To Decimal String(number=w1135) -> (decimal integer string=w1134:string)  [unwired: 1 in]
        n172 = Number To Decimal String(number=w1139) -> (decimal integer string=w1138:string)  [unwired: 1 in]
        n173 = Number To Decimal String(number=w1143) -> (decimal integer string=w1142:string)  [unwired: 1 in]
        n174 = Build Array(w1133, w1129, w1132, w1131, w1130, w1127, w1146, w1145, w1134, w1136, w1137, w1138, w1140, w1141, w1142, w1100, w1101) -> (w1114:string[])
        "appended array 4" <- w1114
        n175 = Insert Into Array(array=w1149, new element=w1114) -> (w1150:string[][])  [unwired: 2 in]
      }
      n176 = call-poly <vilib>:"DB Tools Free Object.vi"("error in (no error)"=w1092, "recordset reference"=w1096) -> ("error out"=w1091:errorcluster, "connection reference"=w1095:T1)  [unwired: 8 in]
      n177 = call <vilib>:"DB Tools Close Connection.vi"("error in (no error)"=w1091, "connection reference"=w1095) -> ("error out"=→"error out 5":errorcluster)  [unwired: 5 in]
      n178 = Array Size(array=w1068) -> ()  [unwired: 1 out]
      n179 = Add Array Elements(numeric array=w1049) -> (sum=w1044:i32)
      n180 = Add Array Elements(numeric array=w1050) -> (sum=w1045:i32)
      n181 = Add Array Elements(numeric array=w1041) -> (sum=w1037:i32)
      n182 = Add Array Elements(numeric array=w1032) -> (sum=w1030:i32)
      n183 = Add Array Elements(numeric array=w1040) -> (sum=w1036:i32)
      n184 = Add Array Elements(numeric array=w1033) -> (sum=w1031:i32)
      n185 = Add Array Elements(numeric array=w1061) -> (sum=w1056:i32)
      n186 = Add Array Elements(numeric array=w1060) -> (sum=w1055:i32)
      n187 = Subtract(x=w1031, y=w1030) -> (x-y=w1029:i32)
      n188 = Subtract(x=w1037, y=w1036) -> (x-y=w1034:i32)
      n189 = Subtract(x=w1056, y=w1055) -> (x-y=w1048:i32)
      n190 = Subtract(x=w1045, y=w1044) -> (x-y=w1042:i32)
      n191 = Number To Decimal String(number=w1044) -> (decimal integer string=w1046:string)  [unwired: 1 in]
      n192 = Number To Decimal String(number=w1042) -> (decimal integer string=w1043:string)  [unwired: 1 in]
      n193 = Number To Decimal String(number=w1037) -> (decimal integer string=w1039:string)  [unwired: 1 in]
      n194 = Number To Decimal String(number=w1036) -> (decimal integer string=w1038:string)  [unwired: 1 in]
      n195 = Number To Decimal String(number=w1034) -> (decimal integer string=w1035:string)  [unwired: 1 in]
      n196 = Number To Decimal String(number=w1029) -> (decimal integer string=w1026:string)  [unwired: 1 in]
      n197 = Number To Decimal String(number=w1056) -> (decimal integer string=w1058:string)  [unwired: 1 in]
      n198 = Number To Decimal String(number=w1055) -> (decimal integer string=w1057:string)  [unwired: 1 in]
      n199 = Number To Decimal String(number=w1045) -> (decimal integer string=w1047:string)  [unwired: 1 in]
      n200 = Number To Decimal String(number=w1031) -> (decimal integer string=w1028:string)  [unwired: 1 in]
      n201 = Number To Decimal String(number=w1030) -> (decimal integer string=w1027:string)  [unwired: 1 in]
      n202 = Number To Decimal String(number=w1048) -> (decimal integer string=w1054:string)  [unwired: 1 in]
      n203 = Build Array(w1059, w1059, "Total :" ("element"), w1058, w1057, w1054, w1047, w1046, w1043, w1039, w1038, w1035, w1028, w1027, w1026, w1024, w1024) -> (w1053:string[])
      n204 = Insert Into Array(array=w1052, new element=w1053) -> (w1051:string[][])  [unwired: 2 in]
      n205 = local write "Table Control 3"(w1051) -> ()
    }
    frame #3 {
      w1535 = ""
      w1570 = ""
      n206 = call-poly <vilib>:"DB Tools Open Connection.vi"("connection information"=path "c:/m100/data/m100.dsn") -> ("error out"=w1605:errorcluster, "connection reference"=w1609:T1)  [unwired: 7 in]
      n207 = call-poly <vilib>:"DB Tools Execute Query.vi"("error in (no error)"=w1605, "SQL query"="select distinct d.mt_customer,d.mt_package,d.mt_device,\n      (select isnull(sum(a.mt_pass),0) from m100.dbo.mt_data a\n      where a.mt_customer=d.mt_customer\n        and a.mt_package=d.mt_package\n        and a.mt_device=d.mt_device\n        and a.mt_machine like 'QAM%'\n        and a.mt_rc_no like 'A%' \n        and CONVERT(varchar,a.mt_end,111)=convert(varchar,getdate()-4,111)\n        and a.mt_shift='©]') as shifta,\n        (select isnull(sum(a.mt_total),0) from m100.dbo.mt_data a\n      where a.mt_customer=d.mt_customer\n        and a.mt_package=d.mt_package\n        and a.mt_device=d.mt_device\n        and a.mt_machine like 'QAM%'\n        and a.mt_rc_no like 'A%' \n        and CONVERT(varchar,a.mt_end,111)=convert(varchar,getdate()-4,111)\n        and a.mt_shift='©]') as shifta1,\n        (select isnull(sum(b.mt_pass),0) from m100.dbo.mt_data b\n      where b.mt_customer=d.mt_customer\n        and b.mt_package=d.mt_package\n       and b.mt_device=d.mt_device\n        and b.mt_machine like 'QAM%'\n        and b.mt_rc_no like 'A%' \n        and CONVERT(varchar,b.mt_end,111)=convert(varchar,getdate()-4,111)\n        and b.mt_shift='¦­') as shiftb,\n        (select isnull(sum(b.mt_total),0) from m100.dbo.mt_data b\n      where b.mt_customer=d.mt_customer\n        and b.mt_package=d.mt_package\n        and b.mt_device=d.mt_device\n        and b.mt_machine like 'QAM%'\n        and b.mt_rc_no like 'A%' \n        and CONVERT(varchar,b.mt_end,111)=convert(varchar,getdate()-4,111)\n        and b.mt_shift='¦­') as shiftb1,\n        (select isnull(sum(c.mt_pass),0) from m100.dbo.mt_data c\n      where c.mt_customer=d.mt_customer\n        and c.mt_package=d.mt_package\n        and c.mt_device=d.mt_device\n        and c.mt_machine like 'QAM%'\n        and c.mt_rc_no like 'A%' \n        and CONVERT(varchar,c.mt_end,111)=convert(varchar,getdate()-4,111)\n        and c.mt_shift='¤¤') as shiftc,\n        (select isnull(sum(c.mt_total),0) from m100.dbo.mt_data c\n      where c.mt_customer=d.mt_customer\n        and c.mt_package=d.mt_package\n        and c.mt_device=d.mt_device\n        and c.mt_machine like 'QAM%'\n        and c.mt_rc_no like 'A%' \n        and CONVERT(varchar,c.mt_end,111)=convert(varchar,getdate()-4,111)\n        and c.mt_shift='¤¤') as shiftc1,\n        SUM(mt_pass),SUM(mt_total),master.dbo.GetEntityNameFromDateToDate(d.mt_customer,d.mt_package,d.mt_device,CONVERT(varchar,GETDATE()-4,111),CONVERT(varchar,GETDATE()-4,111))\n  FROM [m100].[dbo].[mt_data] d\n  WHERE  d.mt_machine like 'QAM%'\n    AND CONVERT(varchar,d.mt_end,111)=convert(varchar,getdate()-4,111)\n    and d.mt_pass > 0 and d.mt_rc_no like 'A%'\n      group by d.mt_customer,d.mt_package,d.mt_device", "connection reference"=w1609) -> ("error out"=w1604:errorcluster, "recordset reference"=w1608:T2)  [unwired: 5 in]
      n208 = call-poly <vilib>:"DB Tools Fetch Recordset Data.vi"("error in (no error)"=w1604, "recordset reference"=w1608) -> ("error out"=w1603:errorcluster, "recordset data"=w1573:variant[][], "recordset reference out"=w1607:T2)  [unwired: 3 in]
      "recordset data 5" <- w1573
      n209 = Index Array(array=w1573, index (col) #1=0 ("index (row)"), index (col) #2=1 ("index (col)"), index (col) #3=2 ("disabled index (col)"), index (col) #4=3 ("index (col)"), index (col) #5=4 ("index (col)"), index (col) #6=5 ("index (col)"), index (col) #7=6 ("index (col)"), index (col) #8=7 ("index (col)"), index (col) #9=8 ("index (col)"), index (col) #10=9 ("index (col)"), index (col) #11=10 ("index (col)"), index (col) #12=11 ("index (col)")) -> (element #1=w1577:variant[], element #2=w1576:variant[], element #3=w1590:variant[], element #4=w1589:variant[], element #5=w1588:variant[], element #6=w1587:variant[], element #7=w1586:variant[], element #8=w1585:variant[], element #9=w1584:variant[], element #10=w1583:variant[], element #11=w1582:variant[], element #12=w1581:variant[])  [unwired: 12 in]
      n210 = for {
        tunnel: w1590 -> [w1635] mode=indexing
        tunnel: w1589 -> [w1634] mode=indexing
        tunnel: w1588 -> [w1633] mode=indexing
        tunnel: w1587 -> [w1632] mode=indexing
        tunnel: w1586 -> [w1631] mode=indexing
        tunnel: w1585 -> [w1630] mode=indexing
        tunnel: w1584 -> [w1629] mode=indexing
        tunnel: w1583 -> [w1628] mode=indexing
        tunnel: w1582 -> [w1627] mode=indexing
        tunnel: w1581 -> [w1626] mode=indexing
        tunnel: [w1661] -> w1563
        shift-right: [w1661] -> w1579
        shift-left: string[][] [] ("array") -> [w1660]
        tunnel: w1577 -> [w1637] mode=indexing
        tunnel: w1576 -> [w1636] mode=indexing
        tunnel: [w1624] -> w1572 mode=indexing
        tunnel: [w1623] -> w1571 mode=indexing
        tunnel: [w1622] -> w1561 mode=indexing
        tunnel: [w1621] -> w1560 mode=indexing
        tunnel: [w1620] -> w1552 mode=indexing
        tunnel: [w1619] -> w1551 mode=indexing
        tunnel: [w1613] -> w1544 mode=indexing
        tunnel: [w1614] -> w1543 mode=indexing
        w1659 = ""
        n211 = xnode "Database Variant To Data"("database variant"=w1634, "type"=0) -> ("data"=w1624:i32)  [unwired: 1 in, 1 out]
        n212 = xnode "Database Variant To Data"("database variant"=w1631, "type"=w1624) -> ("data"=w1621:i32)  [unwired: 1 in, 1 out]
        n213 = xnode "Database Variant To Data"("database variant"=w1628, "type"=w1621) -> ("data"=w1613:i32)  [unwired: 1 in, 1 out]
        n214 = xnode "Database Variant To Data"("database variant"=w1635, "type"=w1659) -> ("data"=w1643:string)  [unwired: 1 in, 1 out]
        n215 = xnode "Database Variant To Data"("database variant"=w1632, "type"=w1624) -> ("data"=w1622:i32)  [unwired: 1 in, 1 out]
        n216 = xnode "Database Variant To Data"("database variant"=w1629, "type"=w1621) -> ("data"=w1619:i32)  [unwired: 1 in, 1 out]
        n217 = xnode "Database Variant To Data"("database variant"=w1626, "type"="") -> ("data"=w1612:string)  [unwired: 1 in, 1 out]
        n218 = xnode "Database Variant To Data"("database variant"=w1630, "type"=w1621) -> ("data"=w1620:i32)  [unwired: 1 in, 1 out]
        n219 = xnode "Database Variant To Data"("database variant"=w1636, "type"=w1659) -> ("data"=w1640:string)  [unwired: 1 in, 1 out]
        n220 = Number To Decimal String(number=w1624) -> (decimal integer string=w1642:string)  [unwired: 1 in]
        n221 = xnode "Database Variant To Data"("database variant"=w1633, "type"=w1624) -> ("data"=w1623:i32)  [unwired: 1 in, 1 out]
        n222 = xnode "Database Variant To Data"("database variant"=w1627, "type"=w1613) -> ("data"=w1614:i32)  [unwired: 1 in, 1 out]
        n223 = xnode "Database Variant To Data"("database variant"=w1637, "type"=w1659) -> ("data"=w1644:string)  [unwired: 1 in, 1 out]
        n224 = Number To Decimal String(number=w1623) -> (decimal integer string=w1641:string)  [unwired: 1 in]
        n225 = Number To Decimal String(number=w1622) -> (decimal integer string=w1657:string)  [unwired: 1 in]
        n226 = Number To Decimal String(number=w1621) -> (decimal integer string=w1656:string)  [unwired: 1 in]
        n227 = Number To Decimal String(number=w1613) -> (decimal integer string=w1651:string)  [unwired: 1 in]
        n228 = Number To Decimal String(number=w1620) -> (decimal integer string=w1647:string)  [unwired: 1 in]
        n229 = Number To Decimal String(number=w1619) -> (decimal integer string=w1648:string)  [unwired: 1 in]
        n230 = Number To Decimal String(number=w1614) -> (decimal integer string=w1652:string)  [unwired: 1 in]
        n231 = Subtract(x=w1624, y=w1623) -> (x-y=w1639:i32)
        n232 = Divide(x=w1614, y=w1613) -> (x/y=w1618:dbl)
        n233 = Number To Decimal String(number=w1639) -> (decimal integer string=w1638:string)  [unwired: 1 in]
        n234 = Subtract(x=w1622, y=w1621) -> (x-y=w1646:i32)
        n235 = Subtract(x=w1620, y=w1619) -> (x-y=w1650:i32)
        n236 = Multiply(x=w1618, y=100.0) -> (x*y=w1616:dbl)
        n237 = Subtract(x=w1613, y=w1614) -> (x-y=w1654:i32)
        n238 = Number To Decimal String(number=w1646) -> (decimal integer string=w1645:string)  [unwired: 1 in]
        n239 = Number To Decimal String(number=w1650) -> (decimal integer string=w1649:string)  [unwired: 1 in]
        n240 = Number To Fractional String(number=w1616, precision (6)=i16 2) -> (F-format string=w1611:string)  [unwired: 2 in]
        n241 = Number To Decimal String(number=w1654) -> (decimal integer string=w1653:string)  [unwired: 1 in]
        n242 = Build Array(w1644, w1640, w1643, w1642, w1641, w1638, w1657, w1656, w1645, w1647, w1648, w1649, w1651, w1652, w1653, w1611, w1612) -> (w1625:string[])
        "appended array 5" <- w1625
        n243 = Insert Into Array(array=w1660, new element=w1625) -> (w1661:string[][])  [unwired: 2 in]
      }
      n244 = call-poly <vilib>:"DB Tools Free Object.vi"("error in (no error)"=w1603, "recordset reference"=w1607) -> ("error out"=w1602:errorcluster, "connection reference"=w1606:T1)  [unwired: 8 in]
      n245 = call <vilib>:"DB Tools Close Connection.vi"("error in (no error)"=w1602, "connection reference"=w1606) -> ("error out"=→"error out 6":errorcluster)  [unwired: 5 in]
      n246 = Array Size(array=w1579) -> ()  [unwired: 1 out]
      n247 = Add Array Elements(numeric array=w1560) -> (sum=w1555:i32)
      n248 = Add Array Elements(numeric array=w1561) -> (sum=w1556:i32)
      n249 = Add Array Elements(numeric array=w1552) -> (sum=w1548:i32)
      n250 = Add Array Elements(numeric array=w1543) -> (sum=w1541:i32)
      n251 = Add Array Elements(numeric array=w1551) -> (sum=w1547:i32)
      n252 = Add Array Elements(numeric array=w1544) -> (sum=w1542:i32)
      n253 = Add Array Elements(numeric array=w1572) -> (sum=w1567:i32)
      n254 = Add Array Elements(numeric array=w1571) -> (sum=w1566:i32)
      n255 = Subtract(x=w1542, y=w1541) -> (x-y=w1540:i32)
      n256 = Subtract(x=w1548, y=w1547) -> (x-y=w1545:i32)
      n257 = Subtract(x=w1567, y=w1566) -> (x-y=w1559:i32)
      n258 = Subtract(x=w1556, y=w1555) -> (x-y=w1553:i32)
      n259 = Number To Decimal String(number=w1555) -> (decimal integer string=w1557:string)  [unwired: 1 in]
      n260 = Number To Decimal String(number=w1553) -> (decimal integer string=w1554:string)  [unwired: 1 in]
      n261 = Number To Decimal String(number=w1548) -> (decimal integer string=w1550:string)  [unwired: 1 in]
      n262 = Number To Decimal String(number=w1547) -> (decimal integer string=w1549:string)  [unwired: 1 in]
      n263 = Number To Decimal String(number=w1545) -> (decimal integer string=w1546:string)  [unwired: 1 in]
      n264 = Number To Decimal String(number=w1540) -> (decimal integer string=w1537:string)  [unwired: 1 in]
      n265 = Number To Decimal String(number=w1567) -> (decimal integer string=w1569:string)  [unwired: 1 in]
      n266 = Number To Decimal String(number=w1566) -> (decimal integer string=w1568:string)  [unwired: 1 in]
      n267 = Number To Decimal String(number=w1556) -> (decimal integer string=w1558:string)  [unwired: 1 in]
      n268 = Number To Decimal String(number=w1542) -> (decimal integer string=w1539:string)  [unwired: 1 in]
      n269 = Number To Decimal String(number=w1541) -> (decimal integer string=w1538:string)  [unwired: 1 in]
      n270 = Number To Decimal String(number=w1559) -> (decimal integer string=w1565:string)  [unwired: 1 in]
      n271 = Build Array(w1570, w1570, "Total :" ("element"), w1569, w1568, w1565, w1558, w1557, w1554, w1550, w1549, w1546, w1539, w1538, w1537, w1535, w1535) -> (w1564:string[])
      n272 = Insert Into Array(array=w1563, new element=w1564) -> (w1562:string[][])  [unwired: 2 in]
      n273 = local write "Table Control 4"(w1562) -> ()
    }
    frame #4 {
      w2066 = "macro1" ("macro name")
      w2140 = "M100DailyThroughput"
      w2082 = string[] ["Customer", "Package", "Device", "Total", "Pass", "Fail", "Total", "Pass", "Fail", "Total", "Pass", "Fail", "Total", "Pass", "Fail", "Yield%", "Machine"] ("row headers")
      w2062 = cluster{"row":i32, "column":i32} {"row"=0, "column"=0} ("end (-1, -1)")
      w2157 = T3."Excel"  # Report Type
      # "Simulate UUT Testing"
      n274 = call <vilib>:"New Report.vi"("report type"=w2157, "template (empty)"="Report Template") -> ("report out"=w2153:refnum<class "NI_report.lvclass">, "error out"=w2152:errorcluster)  [unwired: 12 in]
      n275 = call <vilib>:"Excel Get Worksheet.vi"("report in"=w2153, "worksheet index (0)"=0, "error in (no error)"=w2152) -> ("report out"=w2057:refnum<class "NI_report.lvclass">, "error out"=w2056:errorcluster)  [unwired: 11 in]
      n276 = Get Date/Time In Seconds() -> (seconds since 1Jan1904=w2146:timestamp)
      n277 = Subtract(x=w2146, y=86400) -> (x-y=w2053:timestamp)
      n278 = Format Date/Time String(time format string (%c)="%Y-%m-%d", seconds (now)=w2053) -> (date/time string=w2051:string)  [unwired: 1 in]
      n279 = call <vilib>:"Excel Rename Worksheet.vi"("report in"=w2057, "worksheet name (\"\")"=w2051, "error in (no error)"=w2056) -> ("report out"=w2055:refnum<class "NI_report.lvclass">, "error out"=w2054:errorcluster)  [unwired: 11 in]
      n280 = call-poly <vilib>:"Append Table to Report.vi"("report in"=w2055, "column headers"=w2082, "text data"="Table Control", "error in (no error)"=w2054) -> ("report out"=w2155:refnum<class "NI_report.lvclass">, "error out"=w2154:errorcluster)  [unwired: 8 in, 2 out]
      n281 = Get Date/Time String(seconds (now)=w2053) -> (date string=w2138:string)  [unwired: 2 in, 1 out]
      n282 = call <vilib>:"Excel Insert Cells.vi"("report in"=w2155, "error in (no error)"=w2154) -> ("report out"=w2151:refnum<class "NI_report.lvclass">, "error out"=w2150:errorcluster)  [unwired: 12 in]
      n283 = Concatenate Strings("Date :" ("string"), w2138, "  00:00 - 24:00" ("string")) -> (w2148:string)
      n284 = call <vilib>:"Excel Easy Text.vi"("report in"=w2151, "text"=w2148, "start (-1, -1)"=w2062, "error in (no error)"=w2150) -> ("report out"=w2135:refnum<class "NI_report.lvclass">, "error out"=w2134:errorcluster)  [unwired: 7 in, 3 out]
      n285 = call <vilib>:"Excel Run Macro.vi"("report in"=w2135, "macro name"=w2066, "error in (no error)"=w2134) -> ("report out"=w2133:refnum<class "NI_report.lvclass">, "error out"=w2132:errorcluster)  [unwired: 10 in, 1 out]
      n286 = Get Date/Time In Seconds() -> (seconds since 1Jan1904=w2124:timestamp)
      n287 = call <vilib>:"Excel Get Worksheet.vi"("report in"=w2133, "worksheet index (0)"=1, "error in (no error)"=w2132) -> ("report out"=w2130:refnum<class "NI_report.lvclass">, "error out"=w2129:errorcluster)  [unwired: 11 in]
      n288 = Subtract(x=w2124, y=172800) -> (x-y=w2114:timestamp)
      n289 = Get Date/Time String(seconds (now)=w2114) -> (date string=w2115:string)  [unwired: 2 in, 1 out]
      n290 = call-poly <vilib>:"Append Table to Report.vi"("report in"=w2130, "column headers"=w2082, "text data"="Table Control 2", "error in (no error)"=w2129) -> ("report out"=w2127:refnum<class "NI_report.lvclass">, "error out"=w2126:errorcluster)  [unwired: 8 in, 2 out]
      n291 = call <vilib>:"Excel Insert Cells.vi"("report in"=w2127, "error in (no error)"=w2126) -> ("report out"=w2121:refnum<class "NI_report.lvclass">, "error out"=w2120:errorcluster)  [unwired: 12 in]
      n292 = Format Date/Time String(time format string (%c)="%Y-%m-%d", seconds (now)=w2114) -> (date/time string=w2112:string)  [unwired: 1 in]
      n293 = Concatenate Strings("Date :" ("string"), w2115, "  00:00 - 24:00" ("string")) -> (w2111:string)
      n294 = call <vilib>:"Excel Easy Text.vi"("report in"=w2121, "text"=w2111, "start (-1, -1)"=w2062, "error in (no error)"=w2120) -> ("report out"=w2119:refnum<class "NI_report.lvclass">, "error out"=w2118:errorcluster)  [unwired: 7 in, 3 out]
      n295 = call <vilib>:"Excel Run Macro.vi"("report in"=w2119, "macro name"=w2066, "error in (no error)"=w2118) -> ("report out"=w2117:refnum<class "NI_report.lvclass">, "error out"=w2116:errorcluster)  [unwired: 10 in, 1 out]
      n296 = call <vilib>:"Excel Rename Worksheet.vi"("report in"=w2117, "worksheet name (\"\")"=w2112, "error in (no error)"=w2116) -> ("report out"=w2089:refnum<class "NI_report.lvclass">, "error out"=w2088:errorcluster)  [unwired: 11 in]
      n297 = call <vilib>:"Excel Get Worksheet.vi"("report in"=w2089, "worksheet index (0)"=2, "error in (no error)"=w2088) -> ("report out"=w2109:refnum<class "NI_report.lvclass">, "error out"=w2108:errorcluster)  [unwired: 11 in]
      n298 = Get Date/Time In Seconds() -> (seconds since 1Jan1904=w2103:timestamp)
      n299 = call-poly <vilib>:"Append Table to Report.vi"("report in"=w2109, "column headers"=w2082, "text data"="Table Control 3", "error in (no error)"=w2108) -> ("report out"=w2106:refnum<class "NI_report.lvclass">, "error out"=w2105:errorcluster)  [unwired: 8 in, 2 out]
      n300 = Subtract(x=w2103, y=259200) -> (x-y=w2093:timestamp)
      n301 = Get Date/Time String(seconds (now)=w2093) -> (date string=w2094:string)  [unwired: 2 in, 1 out]
      n302 = call <vilib>:"Excel Insert Cells.vi"("report in"=w2106, "error in (no error)"=w2105) -> ("report out"=w2100:refnum<class "NI_report.lvclass">, "error out"=w2099:errorcluster)  [unwired: 12 in]
      n303 = Concatenate Strings("Date :" ("string"), w2094, "  00:00 - 24:00" ("string")) -> (w2090:string)
      n304 = call <vilib>:"Excel Easy Text.vi"("report in"=w2100, "text"=w2090, "start (-1, -1)"=w2062, "error in (no error)"=w2099) -> ("report out"=w2098:refnum<class "NI_report.lvclass">, "error out"=w2097:errorcluster)  [unwired: 7 in, 3 out]
      n305 = Format Date/Time String(time format string (%c)="%Y-%m-%d", seconds (now)=w2093) -> (date/time string=w2091:string)  [unwired: 1 in]
      n306 = call <vilib>:"Excel Run Macro.vi"("report in"=w2098, "macro name"=w2066, "error in (no error)"=w2097) -> ("report out"=w2096:refnum<class "NI_report.lvclass">, "error out"=w2095:errorcluster)  [unwired: 10 in, 1 out]
      n307 = call <vilib>:"Excel Rename Worksheet.vi"("report in"=w2096, "worksheet name (\"\")"=w2091, "error in (no error)"=w2095) -> ("report out"=w2087:refnum<class "NI_report.lvclass">, "error out"=w2086:errorcluster)  [unwired: 11 in]
      n308 = Get Date/Time In Seconds() -> (seconds since 1Jan1904=w2075:timestamp)
      n309 = call <vilib>:"Excel Get Worksheet.vi"("report in"=w2087, "worksheet index (0)"=3, "error in (no error)"=w2086) -> ("report out"=w2084:refnum<class "NI_report.lvclass">, "error out"=w2083:errorcluster)  [unwired: 11 in]
      n310 = Subtract(x=w2075, y=345600) -> (x-y=w2072:timestamp)
      n311 = Get Date/Time String(seconds (now)=w2072) -> (date string=w2070:string)  [unwired: 2 in, 1 out]
      n312 = Concatenate Strings("Date :" ("string"), w2070, "  00:00 - 24:00" ("string")) -> (w2069:string)
      n313 = call-poly <vilib>:"Append Table to Report.vi"("report in"=w2084, "column headers"=w2082, "text data"="Table Control 4", "error in (no error)"=w2083) -> ("report out"=w2080:refnum<class "NI_report.lvclass">, "error out"=w2079:errorcluster)  [unwired: 8 in, 2 out]
      n314 = call <vilib>:"Excel Insert Cells.vi"("report in"=w2080, "error in (no error)"=w2079) -> ("report out"=w2078:refnum<class "NI_report.lvclass">, "error out"=w2077:errorcluster)  [unwired: 12 in]
      n315 = Format Date/Time String(time format string (%c)="%Y-%m-%d", seconds (now)=w2072) -> (date/time string=w2063:string)  [unwired: 1 in]
      n316 = call <vilib>:"Excel Easy Text.vi"("report in"=w2078, "text"=w2069, "start (-1, -1)"=w2062, "error in (no error)"=w2077) -> ("report out"=w2068:refnum<class "NI_report.lvclass">, "error out"=w2067:errorcluster)  [unwired: 7 in, 3 out]
      n317 = call <vilib>:"Excel Run Macro.vi"("report in"=w2068, "macro name"=w2066, "error in (no error)"=w2067) -> ("report out"=w2065:refnum<class "NI_report.lvclass">, "error out"=w2064:errorcluster)  [unwired: 10 in, 1 out]
      n318 = call "DateTimeToStringDateWith0.vi"("time stamp"=w2053) -> ("Dateyyyymmdd"=w2141:string)  [unwired: 9 in, 1 out]
      n319 = call <vilib>:"Excel Rename Worksheet.vi"("report in"=w2065, "worksheet name (\"\")"=w2063, "error in (no error)"=w2064) -> ("report out"=w2050:refnum<class "NI_report.lvclass">, "error out"=w2048:errorcluster)  [unwired: 11 in]
      n320 = Concatenate Strings(w2140, w2141, ".xls" ("string")) -> (w2142:string)
      n321 = Concatenate Strings(w2140, w2141) -> ()  [unwired: 1 out]
      n322 = call <vilib>:"Excel Get Worksheet.vi"("report in"=w2050, "worksheet index (0)"=0, "error in (no error)"=w2048) -> ("report out"=w2049:refnum<class "NI_report.lvclass">, "error out"=w2047:errorcluster)  [unwired: 11 in]
      n323 = Build Path(base path=path "o:/monitor/report", name or relative path=w2142) -> (appended path=w2139:path)
      n324 = call-dynamic "Save Report to File.vi"("report in"=w2049, "report file path"=w2139, "error in (no error)"=w2047) -> ("report out"=w2059:refnum<class "NI_report.lvclass">, "error out"=w2058:errorcluster)  [unwired: 11 in]
      n325 = call-dynamic "Dispose Report.vi"("report in"=w2059, "save changes? (F)"=FALSE, "error in (no error)"=w2058) -> ("error out"=→"error out 4":errorcluster)  [unwired: 12 in]
    }
    frame #5 {
      n326 = Index Array(array=w2161) -> (element=w2160:i32)  [unwired: 1 in]
      n327 = Greater?(x=w2160, y=1) -> (0:w2158:bool)
      n328 = case shown="True" w2158 {
        tunnel: w2163 -> [_ w2164]
        tunnel: w2162 -> [_ w2165]
        frame False {
        }
        frame True {
          (unwired) string[] ["yyliao@ptse.com.tw", "whlee@ptse.com.tw", "s100@ptse.com.tw", "eric_fan@ptse.com.tw", "saulwang@ptse.com.tw", "jtwu@ptse.com.tw"] ("recipients")
          (unwired) "****M100 Daily Throughput Report *****" ("subject ([No Subject])")
          (unwired) string[] ["yyliao@ptse.com.tw"] ("recipients")
          n329 = Current VI's Path() -> (path=w2170:path)
          n330 = Strip Path(path=w2170) -> (name=w2169:string)  [unwired: 1 out]
          n331 = Match Pattern(string=w2169, regular expression=".vi") -> (before substring=w2167:string)  [unwired: 1 in, 3 out]
          n332 = call "MailMessage.vi"("AddSubject"=w2165, "message"="Dear sirs,\n\nAs subjects, attached the M100 Daily Throughput Report for your information,\n\nBest Regards,\n\n", "file path"=w2164, "program"=w2167) -> ()  [unwired: 8 in]
        }
      }
    }
    frame #6 {
      n333 = Quit LabVIEW() -> ()  [unwired: 1 in]
    }
  }
